vi "main.vi"() -> ()   [LabVIEW 2014]
uses:
  Modules/PmuImpairPlugins/PmuImpairPluginBase_class/TypeDefs/clImpairConfig.ctl
  Framework/FrontPanel/TypeDefs/clEventConfig.ctl
  Framework/FrontPanel/TypeDefs/clFrontPanelControlRefs.ctl
  Framework/FrontPanel/TypeDefs/clFrontPanelButtonRefs.ctl
  Framework/Bus_class/Public/TypeDefs/clBusData.ctl
  Modules/EventPlugins/EventPluginBaseClass/TypeDefs/clEvtReportArray.ctl
  Modules/EventPlugins/EventPluginBaseClass/TypeDefs/clEvtReport.ctl
  Modules/EventPlugins/EventPluginBaseClass/TypeDefs/dblEvtSignalArray.ctl
  Modules/NetworkImpairmentModule/PublicAPI/Arguments/Broadcasts/dblNetworkTime.ctl
  Modules/NetworkImpairmentModule/PublicAPI/Arguments/Broadcasts/dblPktLoss.ctl
  Modules/FlagImpairModule/PublicAPI/Arguments/Broadcasts/ui32FlagImpairmentArray.ctl
  Modules/OutputToFilePlugins/OutputToFileBasePlugin/Typedefs/PmuCfgOpt.ctl
  Framework/Bus_class/Bus.lvclass/Bus.ctl
  Framework/Config_class/Config.lvclass/Config.ctl
  Modules/EventModule/PublicAPI/Arguments/Broadcasts/clDidInit.ctl
  <userlib>/NIST/ModuleAdminLib/ModuleAdmin/ModuleAdmin.lvclass
  Modules/EventModule/PublicAPI/Arguments/Broadcasts/clStatUpdate.ctl
  Modules/EventModule/PublicAPI/Arguments/Broadcasts/clErrorRpt.ctl
  Modules/EventModule/PublicAPI/Arguments/Requests/clStopArgument.ctl
  Modules/PmuImpairModule/PublicAPI/Arguments/Broadcasts/clDidInit.ctl
  Modules/PmuImpairModule/PublicAPI/Arguments/Broadcasts/clStatUpdate.ctl
  Modules/PmuImpairModule/PublicAPI/Arguments/Broadcasts/clErrorRpt.ctl
  Modules/PmuImpairModule/PublicAPI/Arguments/Requests/clStopArgument.ctl
  Modules/NetworkImpairmentModule/PublicAPI/Arguments/Broadcasts/clDidInit.ctl
  Modules/NetworkImpairmentModule/PublicAPI/Arguments/Broadcasts/clStatUpdate.ctl
  Modules/NetworkImpairmentModule/PublicAPI/Arguments/Broadcasts/clErrorRpt.ctl
  Modules/NetworkImpairmentModule/PublicAPI/Arguments/Requests/clStopArgument.ctl
  Modules/FlagImpairModule/PublicAPI/Arguments/Broadcasts/clDidInit.ctl
  Modules/FlagImpairModule/PublicAPI/Arguments/Broadcasts/clStatUpdate.ctl
  Modules/FlagImpairModule/PublicAPI/Arguments/Broadcasts/clErrorRpt.ctl
  Modules/FlagImpairModule/PublicAPI/Arguments/Requests/clStopArgument.ctl
  Modules/AppModule/PublicAPI/Arguments/Broadcasts/clErrorRpt.ctl
  Framework/Bus_class/Accessors/Read AppModuleID.vi
  Framework/Config_class/Accessors/Read PARTF Root Directory.vi
  <vilib>/Utility/error.llb/Error Cluster From Error Code.vi
  <vilib>/ErrorRing/Error Ring.xnode
  Framework/Config_class/Config.lvclass
  Framework/Framework.lvlib
  <userlib>/NIST/NISTErrorLib/NISTErrorLib.lvlib
  Framework/Bus_class/Bus.lvclass
  Modules/EventModule/EventModule.lvlib
  Modules/PmuImpairModule/PmuImpairModule.lvlib
  Modules/NetworkImpairmentModule/NetworkImpairmentModule.lvlib
  Modules/FlagImpairModule/FlagImpairModule.lvlib
  Modules/EventPlugins/EventPluginBaseClass/EventPluginBaseClass.lvclass
  Modules/OutputToFilePlugins/OutputToFileBasePlugin/OutputToFileBasePlugin.lvclass
  Modules/PmuImpairPlugins/PmuImpairPluginBase_class/PmuImpairPluginBase.lvclass
  TestAutomation/Comms/Comms.lvlib
  Modules/AppModule/AppModule.lvlib
  TestAutomation/LV-PY/LV-PY.lvlib
  Framework/BusController/BusController.lvlib
  Modules/OutputToFileModule/OutputToFileModule.lvlib
  <vilib>/Utility/config.llb/NI_LVConfig.lvlib
panel:
  in  "btnScriptPath":bool
  in  "Monte Carlo Script":string="Default.py"
  in  "btnTestPath":bool
  in  "Test File":string="Default.tst"
  in  "ShowPanels?":bool caption="Show Module Panels?"
  in  "chkLeaveCmdOpen":bool caption="Leave Script Window Open for Debugging"
  in  "btnMonteCarlo":bool
  in  "Output File Type":u16(ring) items=["none", "CSV"]
  in  "btnOutToFileConfig":bool
  in  "btnVisualize":bool
  in  "btnOpen":bool
  in  "btnAppConfig":bool
  in  "Application Type":u16(ring) caption="Application" items=["none", "LSE", "Ringdown"]
  in  "Impairments":T1(tab)
  in  "Sensor Impairment Parameters":string[][](table)
  in  "clImpairConfig":T2={"FilterType"="Hamming", "bPosSeq"=TRUE}
  in  "Sensor Impairment Type":u16(ring)=2 items=["C37.118.1 PMU Behaviour", "C37.118.1 PMU DSP Model", "None", "PMU Sine Model", "User Impair Example 1"]
  in  "Network Impairment Type":u16(ring)=1 items=["Network Impairment", "None"]
  in  "Network Impairment Parameters":string[][](table)
  in  "Status Impairment Parameters":string[][](table)
  in  "Status Impairment Type":u16(ring)=2 items=["C37.118.2 PMU Data Transmission", "IEC61850 PMU", "None"]
  in  "Bus Number":u8(ring)
  in  "btnUpdateBus":bool
  in  "btnRemoveBus":bool
  in  "btnAbortMonteCarlo":bool
  in  "btnAddBus":bool
  in  "btnExit":bool
  in  "btnSingleRun":bool
  in  "End Time":dbl=5.0
  in  "Start Time":dbl
  in  "Event Configuration":T3={"UTC Time 0"=timestamp(0 s since 1904-01-01), "Nominal Frequency"=60, "Reporting Rate"=60, "Fsamp"=960, "PosSeq"=TRUE} {"Reporting Rate" items=["10 FPS"=10, "12 FPS"=12, "15 FPS"=15, "20 FPS"=20, "30 FPS"=30, "60 FPS"=60]; "Nominal Frequency" items=["50 Hz"=50, "60 Hz"=60]}
  in  "Event Type":u16(ring) items=["C37.118.1", "Event From CSV", "IEEEBusSystem", "Ringdown", "User1"]
  in  "btnSave":bool
  in  "Event Parameters":string[][](table)=[["70", "70", "70", "20", "20", "20"], ["60", "60", "60", "60", "60", "60"], ["0", "-120", "120", "0", "-120", "120"], ["0", "0", "0", "0", "0", "0"], ["0", "0", "0", "0", "0", "0"], ["0", "0", "0", "0", "0", "0"], ["0", "0", "0", "0", "0", "0"], ["0", "0", "0", "0", "0", "0"], ["0", "0", "0", "0", "0", "0"], ["0", "0", "0", "0", "0", "0"], ["0", "0", "0", "0", "0", "0"], ["0", "0", "0", "0", "0", "0"], ["0", "0", "0", "0", "0", "0"]]
  out "Number of Buses":u8=1 min=1
  in  "btnSettings":bool
  # "The transformer impairment tab will be hidden until\nthe transformer impairment is implemented"
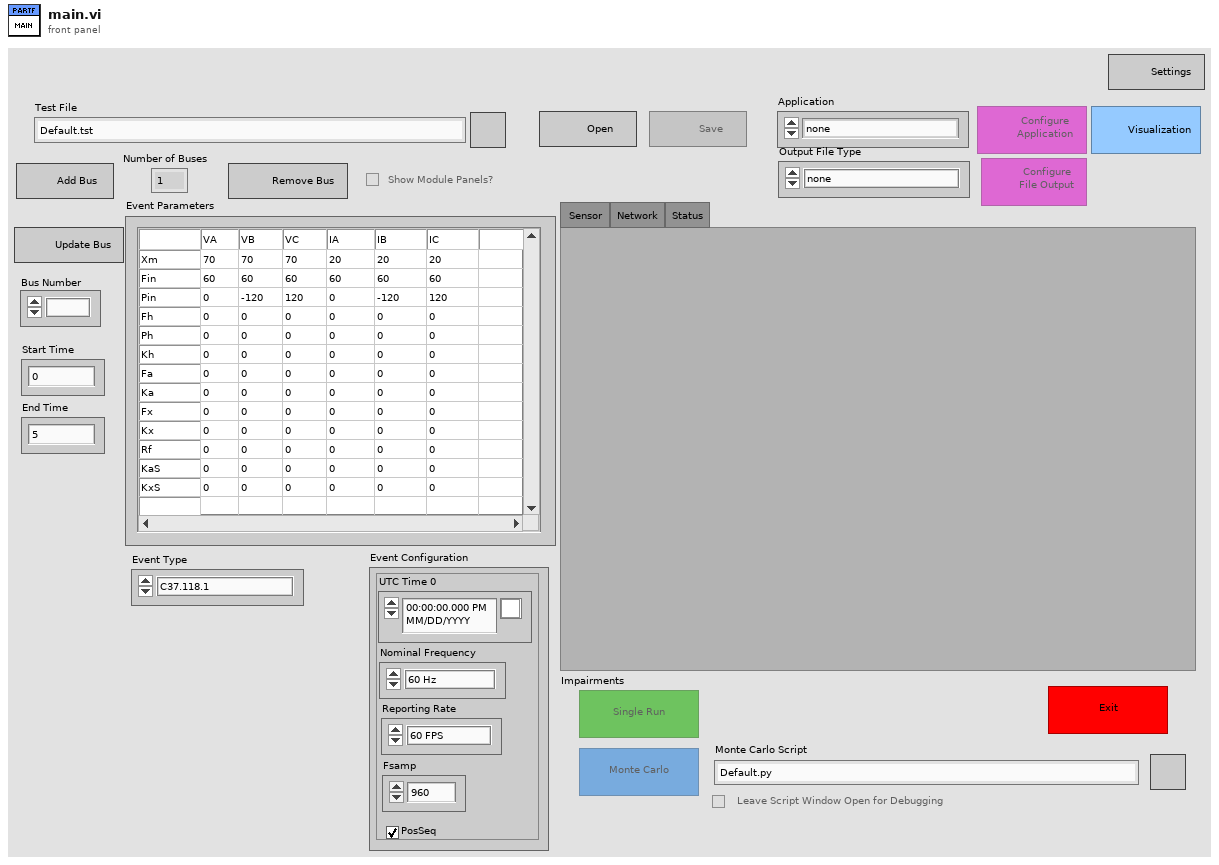
[diagram p1: front panel]
types:
  T1 = enum32{"Transformers", "Sensor ", "Network", "Status"}
  T2 = typedef "PmuImpairPlugins.lvlib/PmuImpairPluginBase.lvclass/clImpairConfig.ctl" = cluster{"FilterType":string, "bPosSeq":bool}
  T3 = typedef "Framework.lvlib/clEventConfig.ctl" = cluster{"UTC Time 0":timestamp, "Nominal Frequency":u16, "Reporting Rate":u16, "Fsamp":u32, "PosSeq":bool}
  T4 = typedef "Framework.lvlib/clFrontPanelButtonRefs.ctl" = cluster{"SaveRef":refnum<vi>, "SingleRunRef":refnum<vi>, "MonteCarloRef":refnum<vi>, "AppConfigRef":refnum<vi>, "chkScriptWindowRef":refnum<vi>, "btnOutToFileConfig":refnum<vi>, "AppTypeRef":refnum<vi>, "chkShowPanel":refnum<vi>}
  T5 = typedef "Framework.lvlib/clFrontPanelControlRefs.ctl" = cluster{"TestFilePathRef":refnum<vi>, "BusNumberRef":refnum<vi>, "NumberOfBusesRef":refnum<vi>, "EvtTypeRef":refnum<vi>, "EvtParamsRef":refnum<vi>, "EvtConfigRef":refnum<vi>, "StartTimeRef":refnum<vi>, "EndTimeRef":refnum<vi>, "PmuImpairTypeRef":refnum<vi>, "PmuImpairParamsRef":refnum<vi>, "NetImpairParamsRef":refnum<vi>, "FlagImpairTypeRef":refnum<vi>, "FlagImpairParamsRef":refnum<vi>, "NetImpairTypeRef":refnum<vi>, "OutputFileType":refnum<vi>, "PmuImpairConfigRef":refnum<vi>, "AppTypeRef":refnum<vi>, "ScriptPathRef":refnum<vi>, "ShowPanels?":refnum<vi>}
  T6 = typedef "EventModule.lvlib/clBroadcastEvents.ctl" = cluster{"DidInit":refnum<user-event>, "StatusUpdate":refnum<user-event>, "ErrorReport":refnum<user-event>, "DidStop":refnum<user-event>, "ReadEvtConfig":refnum<user-event>, "ReadTimeArray":refnum<user-event>, "ReadEvtParams":refnum<user-event>, "GetEvtReportArray":refnum<user-event>, "ReadPathToPlugin":refnum<user-event>, "GetEvtSignal":refnum<user-event>, "ReadBusNumber":refnum<user-event>}
  T7 = typedef "PmuImpairModule.lvlib/clBroadcastEvents.ctl" = cluster{"DidInit":refnum<user-event>, "StatusUpdate":refnum<user-event>, "ErrorReport":refnum<user-event>, "DidStop":refnum<user-event>, "ImpairConfig":refnum<user-event>, "ImpairParams":refnum<user-event>, "ImpairReports":refnum<user-event>, "PathToPlugin":refnum<user-event>, "BusNumber":refnum<user-event>}
  T8 = typedef "NetworkImpairmentModule.lvlib/clBroadcastEvents.ctl" = cluster{"DidInit":refnum<user-event>, "StatusUpdate":refnum<user-event>, "ErrorReport":refnum<user-event>, "DidStop":refnum<user-event>, "ReadNetImpParams":refnum<user-event>, "ReadLossThreshold":refnum<user-event>, "GetNetworkTime":refnum<user-event>, "GetPktLoss":refnum<user-event>, "ReadPathToPlugin":refnum<user-event>}
  T9 = typedef "FlagImpairModule.lvlib/clBroadcastEvents.ctl" = cluster{"DidInit":refnum<user-event>, "StatusUpdate":refnum<user-event>, "ErrorReport":refnum<user-event>, "DidStop":refnum<user-event>, "ReadFlagImpairConfig":refnum<user-event>, "ReadPluginINIFilePath":refnum<user-event>, "ReadFlagImpairParams":refnum<user-event>, "ReadTimeArray":refnum<user-event>, "GetFlagImpairment":refnum<user-event>}
  T10 = typedef "AppModule.lvlib/clBroadcastEvents.ctl" = cluster{"DidInit":refnum<user-event>, "StatusUpdate":refnum<user-event>, "ErrorReport":refnum<user-event>, "DidStop":refnum<user-event>, "PathToINI":refnum<user-event>, "InputData":refnum<user-event>, "OutputData":refnum<user-event>, "BcAppInfo":refnum<user-event>, "ConfigData":refnum<user-event>}
  T11 = typedef "OutputToFileModule.lvlib/clBroadcastEvents.ctl" = cluster{"DidInit":refnum<user-event>, "StatusUpdate":refnum<user-event>, "ErrorReport":refnum<user-event>, "DidStop":refnum<user-event>, "PathToPlugin":refnum<user-event>, "PmuConfig":refnum<user-event>, "OutputPath":refnum<user-event>}
  T12 = typedef "Framework.lvlib/clRequestEvents.ctl" = cluster{"StopRequest":refnum<user-event>}
  T13 = typedef "EventModule.lvlib/clDidInit.ctl" = cluster{"Init?":bool, "ModuleAdmin":refnum<class "ModuleAdmin.lvclass">}
  T14 = typedef "EventModule.lvlib/clStatUpdate.ctl" = cluster{"Status":string}
  T15 = typedef "EventModule.lvlib/clErrorRpt.ctl" = cluster{"error":errorcluster, "AdditionalInfo":string}
  T16 = typedef "EventModule.lvlib/clStopArgument.ctl" = cluster{"Exit via Stop Module Req?":bool, "Wait for Module to stop?":bool, "ModuleAdmin":refnum<class "ModuleAdmin.lvclass">}
  T17 = typedef "PmuImpairModule.lvlib/clDidInit.ctl" = cluster{"Init?":bool, "ModuleAdmin":refnum<class "ModuleAdmin.lvclass">}
  T18 = typedef "PmuImpairModule.lvlib/clStatUpdate.ctl" = cluster{"Status":string}
  T19 = typedef "PmuImpairModule.lvlib/clErrorRpt.ctl" = cluster{"error":errorcluster, "AdditionalInfo":string}
  T20 = typedef "PmuImpairModule.lvlib/clStopArgument.ctl" = cluster{"Exit via Stop Module Req?":bool, "Wait for Module to stop?":bool, "ModuleAdmin":refnum<class "ModuleAdmin.lvclass">}
  T21 = typedef "NetworkImpairmentModule.lvlib/clDidInit.ctl" = cluster{"Init?":bool, "ModuleAdmin":refnum<class "ModuleAdmin.lvclass">}
  T22 = typedef "NetworkImpairmentModule.lvlib/clStatUpdate.ctl" = cluster{"Status":string}
  T23 = typedef "NetworkImpairmentModule.lvlib/clErrorRpt.ctl" = cluster{"error":errorcluster, "AdditionalInfo":string}
  T24 = typedef "NetworkImpairmentModule.lvlib/clStopArgument.ctl" = cluster{"Exit via Stop Module Req?":bool, "Wait for Module to stop?":bool, "ModuleAdmin":refnum<class "ModuleAdmin.lvclass">}
  T25 = typedef "FlagImpairModule.lvlib/clDidInit.ctl" = cluster{"Init?":bool, "ModuleAdmin":refnum<class "ModuleAdmin.lvclass">}
  T26 = typedef "FlagImpairModule.lvlib/clStatUpdate.ctl" = cluster{"Status":string}
  T27 = typedef "FlagImpairModule.lvlib/clErrorRpt.ctl" = cluster{"error":errorcluster, "AdditionalInfo":string}
  T28 = typedef "FlagImpairModule.lvlib/clStopArgument.ctl" = cluster{"Exit via Stop Module Req?":bool, "Wait for Module to stop?":bool, "ModuleAdmin":refnum<class "ModuleAdmin.lvclass">}
  T29 = typedef "AppModule.lvlib/clErrorRpt.ctl" = cluster{"error":errorcluster, "AdditionalInfo":string}
  T30 = typedef "Framework.lvlib/clFrameworkData.ctl" = cluster{"EvtINIFilePaths":path[], "BusClassInstances":refnum<class "Bus.lvclass">[], "PmuImpairINIFilePaths":path[], "FlagImpairINIFilePaths":path[], "NetImpairINIFilePaths":path[], "OutputToFileINIFilePaths":path[], "AppINIFilePaths":path[], "AppModuleID":i32, "OutputToFileID":i32}
  T31 = cluster{"EvtBroadcastEvents":T6, "PmuBroadcastEvents":T7, "NetBroadcastEvents":T8, "FlagImpairBroadcast":T9}
  T32 = typedef "Bus_class.lvlib/Bus.lvclass/clBusData.ctl" = cluster{"BusNumber":u8, "EvtPluginINIFilePath":path, "EvtParams":string[][], "EvtConfig":T3, "Start Time":dbl, "End Time":dbl, "PmuImpairPluginINIFilePath":path, "PmuImpairParams ":string[][], "PmuImpairConfig":T2, "NetImpPluginINIFilePath":path, "NetImpParams":string[][], "FlagImpPluginINIFilePath":path, "FlagImpParams":string[][], "EvtReportArray":T33, "EventSignalArray":T35, "ImpairReportArray":T33, "NetworkTime":T36, "PktLoss":T37, "FlagImpArray":T38, "OutputToFilePluginINIFilePath":path, "Output File Path":path, "clConfigOptions":T39, "AppPluginINIFilePath":path, "AppConfig":variant, "AppOutput":variant}
  T33 = typedef "EventPlugins.lvlib/EventPluginBaseClass.lvclass/clEvtReportArray.ctl" = T34[]
  T34 = typedef "EventPlugins.lvlib/EventPluginBaseClass.lvclass/clEvtReport.ctl" = cluster{"Timestamp":dbl, "Synx":cdb[], "Freq":dbl, "ROCOF":dbl, "ID":i16}
  T35 = typedef "EventPlugins.lvlib/EventPluginBaseClass.lvclass/dblEvtSignalArray.ctl" = dbl[][]
  T36 = typedef "NetworkImpairmentModule.lvlib/dblNetworkTime.ctl" = dbl[]
  T37 = typedef "NetworkImpairmentModule.lvlib/dblPktLoss.ctl" = dbl[]
  T38 = typedef "FlagImpairModule.lvlib/ui32FlagImpairmentArray.ctl" = u32[]
  T39 = typedef "OutputToFilePlugins.lvlib/OutputToFileBasePlugin.lvclass/PmuCfgOpt.ctl" = cluster{"TIME_BASE":u64, "STN":string, "IDCODE":u16, "rdoPolRect":enum32{"Rectangular", "Polar"}, "rdoFloatInt":enum32{"Float", "Integer"}, "PHUNIT":u64, "rdoFreqDfreq":enum32{"Float", "Integer"}, "CHNAM":string[], "chkCfg2Prefix":bool}
  T40 = typedef "NI_LVConfig.lvlib/Config Data RefNum.ctl" = refnum<k1>
  T41 = typedef "AppModule.lvlib/BC_AppInfo.ctl" = cluster{"QueName":string, "BCRegRef":refnum<data-value>}
  T42 = typedef "Framework.lvlib/Config.lvclass/RootDir.ctl" = cluster{"pathRootDir":path, "btnOutPath":bool, "OutDir":string, "btnOpenOutputDir":bool, "ScriptDir":string, "btnOpenScriptDir":bool, "TestDir":string, "btnOpenTestDir":bool}
  T43 = enum8{"Enabled", "Disabled", "Disabled and Grayed Out"}
  T44 = typedef "Framework.lvlib/QueRef.ctl" = refnum<queue>
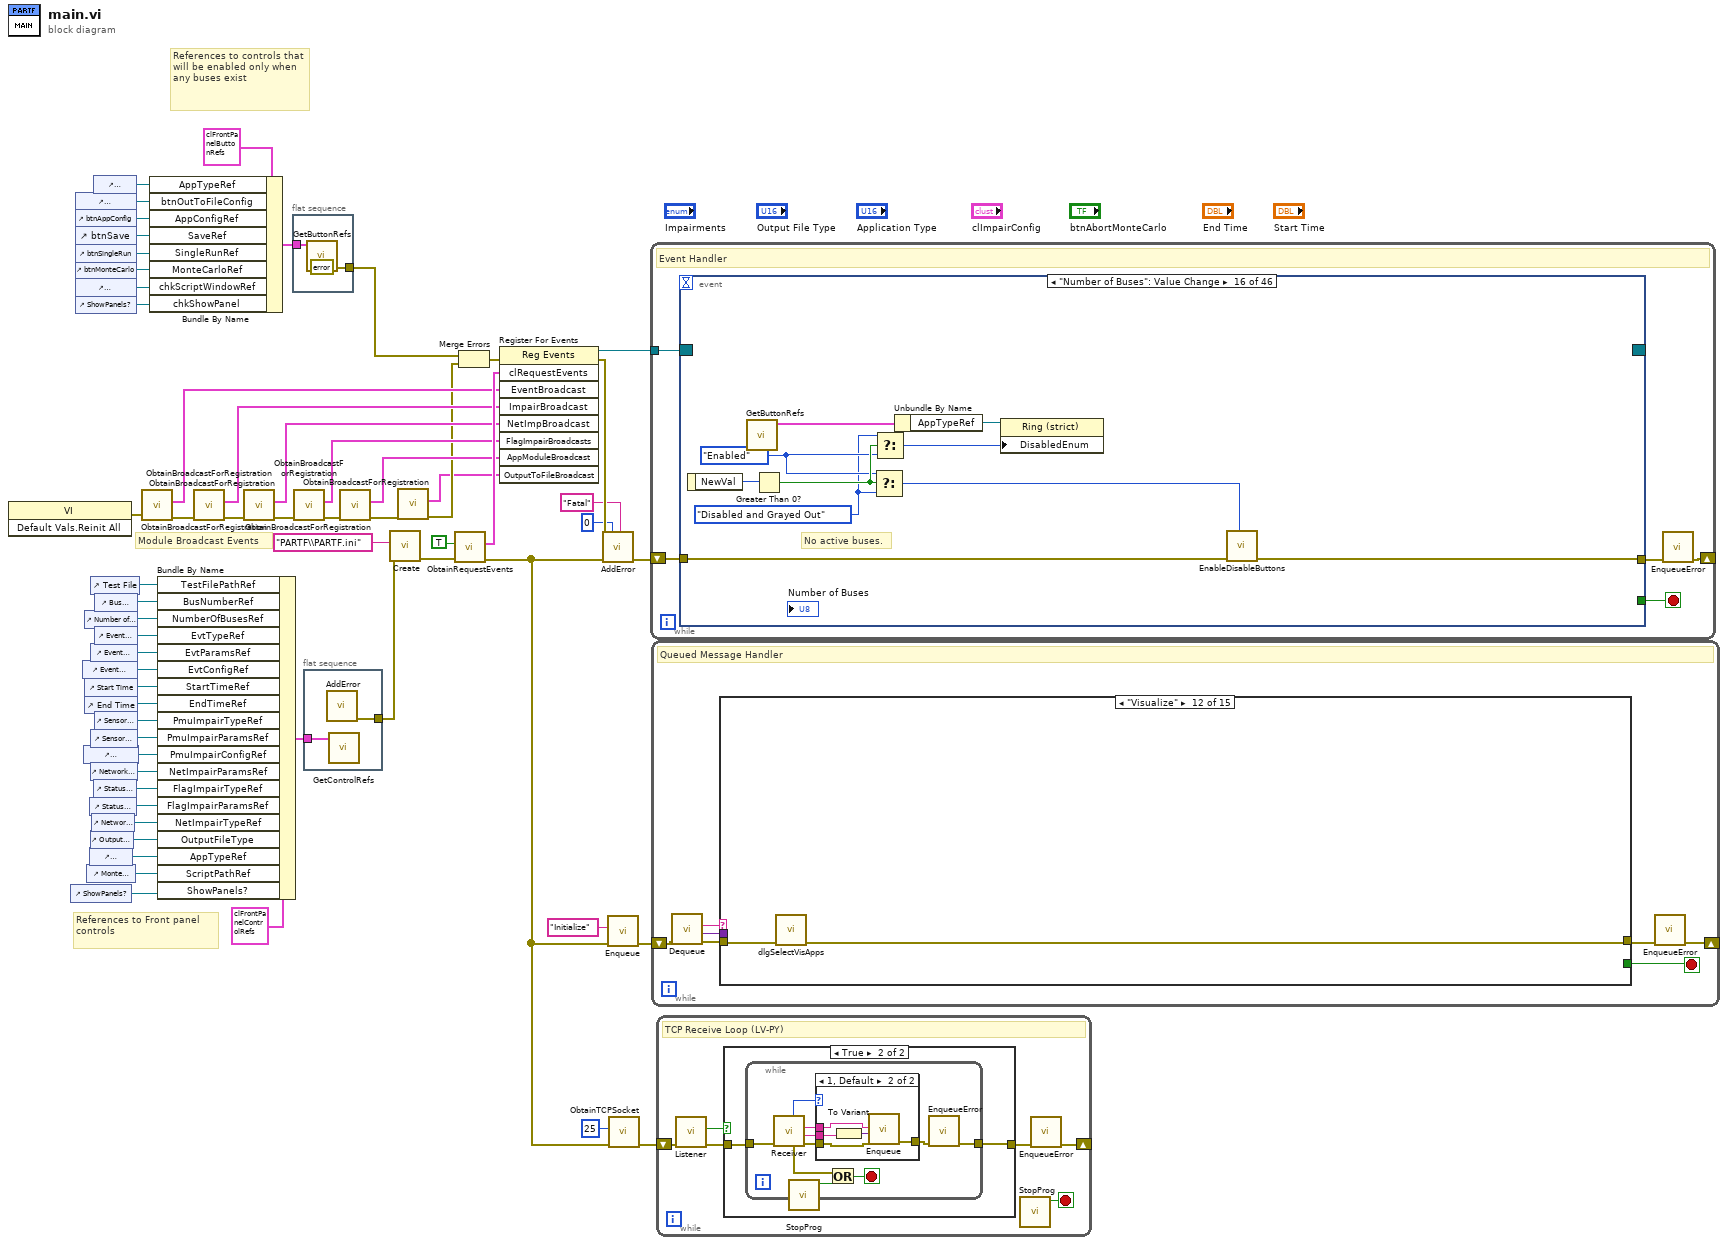
[diagram p0: block diagram]
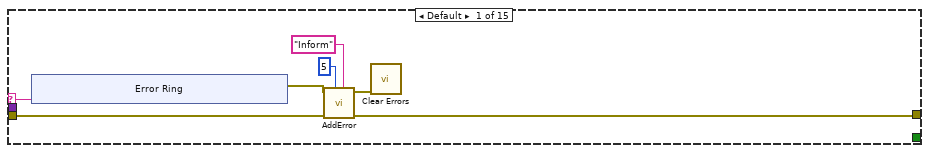
[diagram p4: hidden frame]
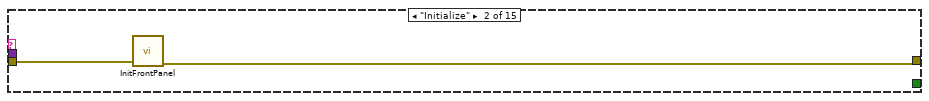
[diagram p5: hidden frame]
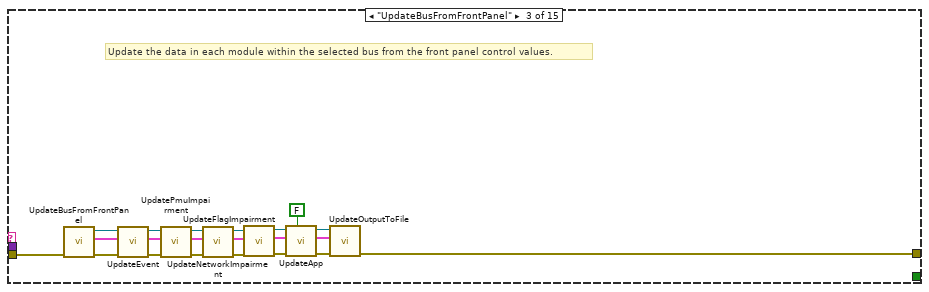
[diagram p6: hidden frame]
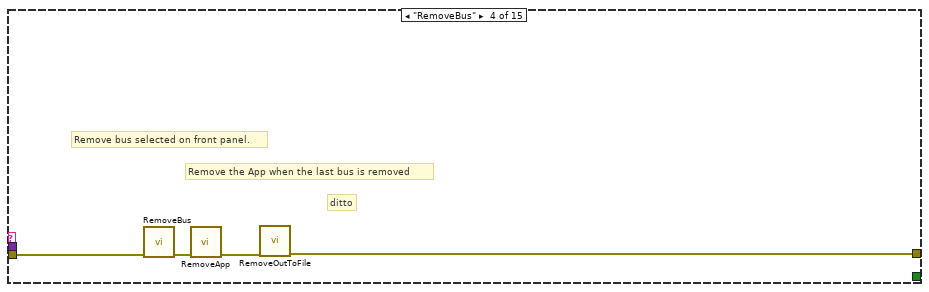
[diagram p7: hidden frame]
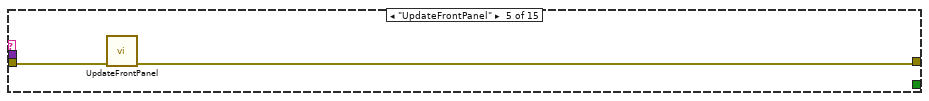
[diagram p8: hidden frame]
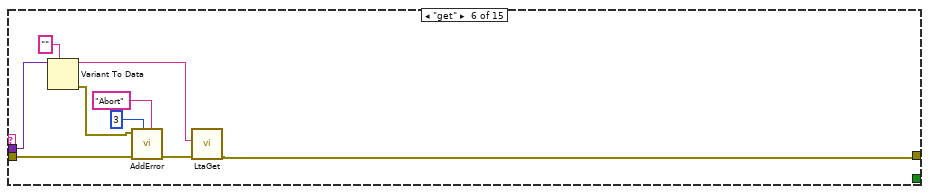
[diagram p9: hidden frame]
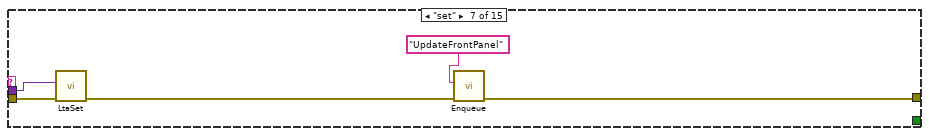
[diagram p10: hidden frame]
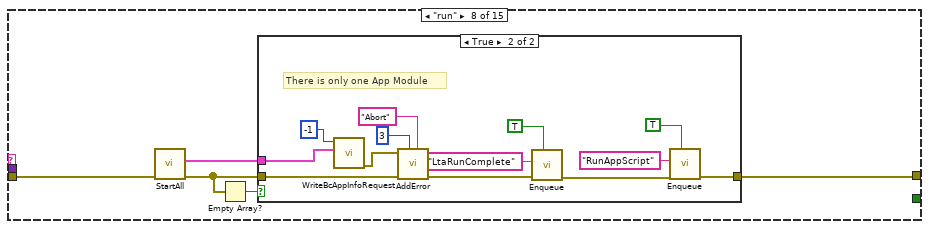
[diagram p11: hidden frame]
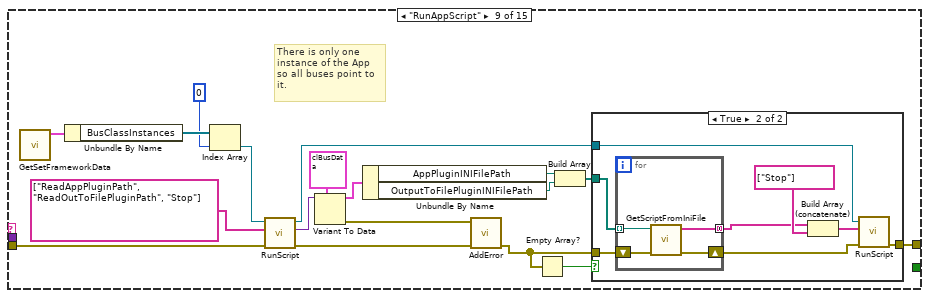
[diagram p13: hidden frame]
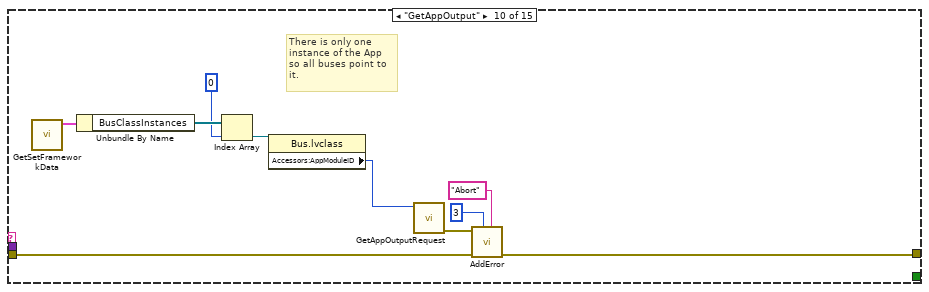
[diagram p15: hidden frame]
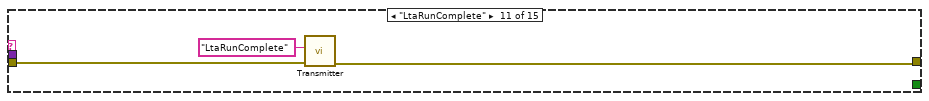
[diagram p16: hidden frame]
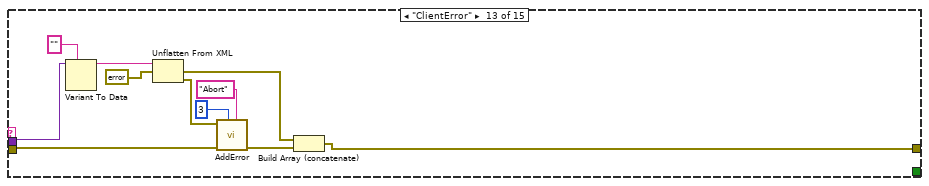
[diagram p17: hidden frame]
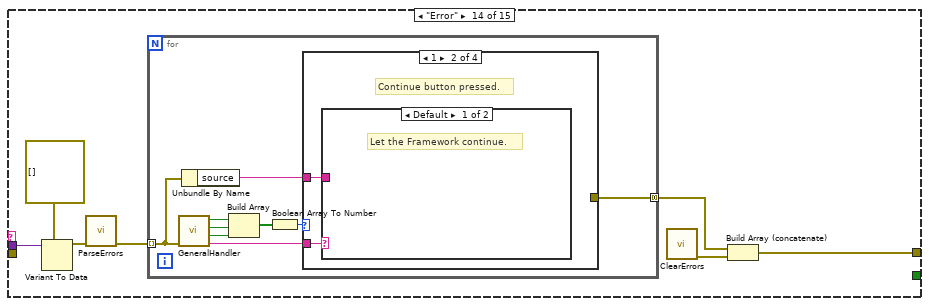
[diagram p18: hidden frame]
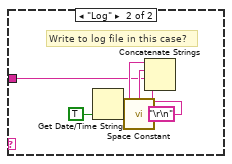
[diagram p20: hidden frame]
diagram:
  # "References to Front panel controls"
  # "Module Broadcast Events"
  # "References to controls that will be enabled only when any buses exist"
  n1 = invoke class="VI" method="Default Vals.Reinit All"() -> (error out=w4:errorcluster)  [unwired: 3 in, 2 out]
  n2 = control-ref of="ShowPanels?"() -> (w10:refnum<vi>)
  n3 = control-ref of="btnOutToFileConfig"() -> (w17:refnum<vi>)
  n4 = control-ref of="btnAppConfig"() -> (w21:refnum<vi>)
  n5 = control-ref of="btnSave"() -> (w46:refnum<vi>)
  n6 = control-ref of="btnSingleRun"() -> (w45:refnum<vi>)
  n7 = control-ref of="btnMonteCarlo"() -> (w44:refnum<vi>)
  n8 = control-ref of="chkLeaveCmdOpen"() -> (w20:refnum<vi>)
  n9 = control-ref of="ShowPanels?"() -> (w9:refnum<vi>)
  n10 = control-ref of="Event Configuration"() -> (w37:refnum<vi>)
  n11 = control-ref of="clImpairConfig"() -> (w24:refnum<vi>)
  n12 = control-ref of="Number of Buses"() -> (w34:refnum<vi>)
  n13 = control-ref of="Start Time"() -> (w33:refnum<vi>)
  n14 = control-ref of="End Time"() -> (w32:refnum<vi>)
  n15 = control-ref of="Monte Carlo Script"() -> (w12:refnum<vi>)
  n16 = control-ref of="Status Impairment Parameters"() -> (w40:refnum<vi>)
  n17 = control-ref of="Application Type"() -> (w13:refnum<vi>)
  n18 = control-ref of="Test File"() -> (w39:refnum<vi>)
  n19 = control-ref of="Event Parameters"() -> (w36:refnum<vi>)
  n20 = control-ref of="Sensor Impairment Parameters"() -> (w54:refnum<vi>)
  n21 = control-ref of="Network Impairment Parameters"() -> (w48:refnum<vi>)
  n22 = control-ref of="Output File Type"() -> (w25:refnum<vi>)
  n23 = control-ref of="Network Impairment Type"() -> (w26:refnum<vi>)
  n24 = control-ref of="Application Type"() -> (w11:refnum<vi>)
  n25 = control-ref of="Status Impairment Type"() -> (w41:refnum<vi>)
  n26 = control-ref of="Bus Number"() -> (w38:refnum<vi>)
  n27 = control-ref of="Event Type"() -> (w35:refnum<vi>)
  n28 = control-ref of="Sensor Impairment Type"() -> (w31:refnum<vi>)
  n29 = call "ObtainBroadcastForRegistration.vi"("error in (no error)"=w4) -> ("error out"=w52:errorcluster, "EventBroadcast"=w53:T6)  [unwired: 9 in]
  n30 = Bundle By Name(cluster=T4 {"SaveRef"=refnum, "SingleRunRef"=refnum, "MonteCarloRef"=refnum, "AppConfigRef"=refnum, "chkScriptWindowRef"=refnum, "btnOutToFileConfig"=refnum, "AppTypeRef"=refnum, "chkShowPanel"=refnum} ("clFrontPanelButtonRefs"), "AppTypeRef"=w11, "btnOutToFileConfig"=w17, "AppConfigRef"=w21, "SaveRef"=w46, "SingleRunRef"=w45, "MonteCarloRef"=w44, "chkScriptWindowRef"=w20, "chkShowPanel"=w9) -> (w3:T4)
  n31 = Bundle By Name(cluster=T5 {"TestFilePathRef"=refnum, "BusNumberRef"=refnum, "NumberOfBusesRef"=refnum, "EvtTypeRef"=refnum, "EvtParamsRef"=refnum, "EvtConfigRef"=refnum, "StartTimeRef"=refnum, "EndTimeRef"=refnum, "PmuImpairTypeRef"=refnum, "PmuImpairParamsRef"=refnum, "NetImpairParamsRef"=refnum, "FlagImpairTypeRef"=refnum, "FlagImpairParamsRef"=refnum, "NetImpairTypeRef"=refnum, "OutputFileType"=refnum, "PmuImpairConfigRef"=refnum, "AppTypeRef"=refnum, "ScriptPathRef"=refnum, "ShowPanels?"=refnum} ("clFrontPanelControlRefs"), "TestFilePathRef"=w39, "BusNumberRef"=w38, "NumberOfBusesRef"=w34, "EvtTypeRef"=w35, "EvtParamsRef"=w36, "EvtConfigRef"=w37, "StartTimeRef"=w33, "EndTimeRef"=w32, "PmuImpairTypeRef"=w31, "PmuImpairParamsRef"=w54, "PmuImpairConfigRef"=w24, "NetImpairParamsRef"=w48, "FlagImpairTypeRef"=w41, "FlagImpairParamsRef"=w40, "NetImpairTypeRef"=w26, "OutputFileType"=w25, "AppTypeRef"=w13, "ScriptPathRef"=w12, "ShowPanels?"=w10) -> (w8:T5)
  n32 = call "ObtainBroadcastForRegistration.vi"("error in (no error)"=w52) -> ("error out"=w50:errorcluster, "ImpairBroadcast"=w51:T7)  [unwired: 9 in]
  n33 = call "ObtainBroadcastForRegistration.vi"("error in (no error)"=w50) -> ("error out"=w43:errorcluster, "NetImpBroadcast"=w49:T8)  [unwired: 9 in]
  n34 = flat-sequence {
    tunnel: w3 -> [w63]
    tunnel: [errorcluster {"status"=FALSE, "code"=0, "source"=""} ("error constant")] -> w1
    frame #0 {
      n35 = call "GetButtonRefs.vi"("BtnRefs"=w63) -> ()  [unwired: 10 in, 1 out]
    }
  }
  n36 = call "ObtainBroadcastForRegistration.vi"("error in (no error)"=w43) -> ("error out"=w19:errorcluster, "FlagImpairBroadcasts"=w42:T9)  [unwired: 9 in]
  n37 = flat-sequence {
    tunnel: w8 -> [w64]
    tunnel: [w65] -> w6
    frame #0 {
      n38 = call <userlib>:"AddError.vi"() -> ("ErrorArray"=w65:errorcluster[])  [unwired: 10 in, 1 out]
      n39 = call "GetControlRefs.vi"("clControlRefs In"=w64) -> ()  [unwired: 10 in, 1 out]
    }
  }
  n40 = call "ObtainBroadcastForRegistration.vi"("error in (no error)"=w19) -> ("error out"=w16:errorcluster, "AppModuleBroadcast"=w18:T10)  [unwired: 9 in]
  n41 = call "Create.vi"("ErrorArray"=w6, "name or relative path"="PARTF\\PARTF.ini") -> ("ErrorArray"=w5:errorcluster[])  [unwired: 8 in, 1 out]
  n42 = call "ObtainBroadcastForRegistration.vi"("error in (no error)"=w16) -> ("error out"=w15:errorcluster, "OutputToFileBroadcast"=w14:T11)  [unwired: 9 in]
  n43 = call "ObtainRequestEvents.vi"("ErrorArray In"=w5, "CreateNew (F)"=TRUE) -> ("ErrorArray Out"=w55:errorcluster[], "clRequestEvents"=w59:T12)  [unwired: 8 in]
  n44 = Merge Errors(w1, w15) -> (w2:errorcluster)
  n45 = register-events(error in=w2, w59, w53, w51, w49, w42, w18, w14) -> (reference out=w58:refnum<event-registration>, error out=w29:errorcluster)  [unwired: 1 in]
  n46 = call <userlib>:"AddError.vi"("Severity"="Fatal" ("String"), "Priority"=u8 0, "ErrorArray"=w55, "error in (no error)"=w29) -> ("ErrorArray"=w30:errorcluster[])  [unwired: 6 in, 1 out]
  n47 = call "Enqueue.vi"("ErrorArray"=w5, "Msg"="Initialize") -> ("ErrorArray"=w61:errorcluster[])  [unwired: 9 in]
  n48 = call "ObtainTCPSocket.vi"("ErrorArray"=w5, "timeout"=25) -> ("ErrorArray"=w23:errorcluster[])  [unwired: 8 in, 1 out]
  n49 = while {
    shift-right: [w67] -> _
    shift-left: w30 -> [w69]
    tunnel: w58 -> [w66]
    stop <- w70 stop-if-true
    # "Event Handler"
    n50 = event shown="[15] \"Number of Buses\": Value Change" {
      selector: w66 -> [_ _ _ w125 _ _ _ w164 _ _ _ _ _ _ _ _ _ _ _ _ _ _ _ _ _ _ _ _ _ _ _ _ _ _ _ _ _ _ _ _ _ _ _ _ _ _]
      dyn-events: [_ _ _ w124 _ _ _ w163 _ _ _ _ _ _ _ _ _ _ _ _ _ _ _ _ _ _ _ _ _ _ _ _ _ _ _ _ _ _ _ _ _ _ _ _ _ _] -> _
      timeout: _ -> [_ _ _ _ _ _ _ _ _ _ _ _ _ _ _ _ _ _ _ _ _ _ _ _ _ _ _ _ _ _ _ _ _ _ _ _ _ _ _ _ _ _ _ _ _ _]
      tunnel: [TRUE _ _ _ _ _ _ _ _ _ _ _ _ _ _ _ _ _ _ _ _ _ _ _ _ _ _ _ TRUE _ _ _ _ _ _ _ _ _ _ _ _ _ _ _ _ _] -> w70
      tunnel: w69 -> [w78 w81 w86 w115 w138 w148 w153 w165 w221 w225 _ w252 w276 _ w305 w315 w318 w322 w324 w326 w328 w331 _ _ w350 w355 w360 w363 w366 w374 w395 w409 w420 w443 w462 w478 w489 w509 w530 w548 w556 w577 w597 w615 w625 w646]
      tunnel: [w77 w80 w85 w96 w139 w151 w152 w162 w220 w226 _ w255 w279 w301 w304 w314 w317 w321 w323 w325 w327 w330 _ _ w349 w351 w356 w362 w365 w373 w393 w410 w422 w442 w464 w479 w491 w507 w529 w546 w557 w576 w599 w617 w626 w648] -> w68
      event "btnExit": Value Change {
        n51 = event-data() -> ()  [unwired: 1 in, 1 out]
        n52 = call "RemoveBus.vi"("Remove All? (F)"=TRUE, "ErrorArray In"=w78) -> ("ErrorArray Out"=w73:errorcluster[])  [unwired: 9 in]
        n53 = call "RemoveApp.vi"("ErrorArray In"=w73) -> ("ErrorArray Out"=w71:errorcluster[])  [unwired: 10 in]
        n54 = call "RemoveOutToFile.vi"("ErrorArray In"=w71) -> ("ErrorArray Out"=w72:errorcluster[])  [unwired: 10 in]
        n55 = call "Enqueue.vi"("Priority (f)"=TRUE, "ErrorArray"=w72, "Msg"="Stop") -> ("ErrorArray"=w77:errorcluster[])  [unwired: 8 in]
      }
      event "btnSettings": Value Change {
        n56 = event-data() -> ()  [unwired: 1 in, 1 out]
        n57 = call "Settings.vi"("ErrorArray"=w81) -> ("ErrorArray"=w80:errorcluster[])  [unwired: 10 in]
      }
      event "btnOutToFileConfig": Value Change {
        n58 = event-data() -> ()  [unwired: 1 in, 1 out]
        n59 = call "GetSetFrameworkData.vi"() -> ("clFrameworkData Out"=w88:T30)  [unwired: 11 in]
        n60 = Unbundle By Name(w88) -> ("OutputToFileID"=w87:i32)
        n61 = call "OpenConfigRequest.vi"("ModuleID"=w87) -> ("error out"=w84:errorcluster)  [unwired: 10 in]
        n62 = call <userlib>:"AddError.vi"("Severity"="Inform", "Priority"=u8 4, "ErrorArray"=w86, "error in (no error)"=w84) -> ("ErrorArray"=w85:errorcluster[])  [unwired: 6 in, 1 out]
      }
      event "btnAddBus": Value Change {
        n63 = event-data() -> ()  [unwired: 1 in, 1 out]
        n64 = property on="ShowPanels?" class="Bool (strict)"() -> ("Value"=w89:bool)  [unwired: 2 in, 2 out]
        n65 = call "Create.vi"("Error In"=w115) -> ("Error Out"=w120:errorcluster[], "Bus out"=w119:refnum<class "Bus.lvclass">)  [unwired: 9 in]
        n66 = call "AddBus.vi"("ShowPanels?"=w89, "ErrorArray In"=w120, "BusClass In"=w119) -> ("ErrorArray Out"=w123:errorcluster[], "UserEvents"=w117:T31, "BusClass Out"=w122:refnum<class "Bus.lvclass">)  [unwired: 6 in]
        n67 = call "AddApp.vi"("ErrorArray In"=w123, "BusClass In"=w122) -> ("ErrorArray Out"=w95:errorcluster[], "clBroadcastEvents"=w121:T10, "BusClass Out"=w93:refnum<class "Bus.lvclass">)  [unwired: 7 in]
        n68 = call "AddOutToFile.vi"("ErrorArray In"=w95, "BusClass In"=w93) -> ("ErrorArray Out"=w94:errorcluster[], "clBroadcastEvents"=w91:T11, "BusClass Out"=w92:refnum<class "Bus.lvclass">)  [unwired: 7 in]
        n69 = Empty Array?(array=w94) -> (empty?=w116:bool)
        n70 = call "InsertBus.vi"("ErrorArray In"=w94, "BusClass In"=w92) -> ("ErrorArray Out"=w118:errorcluster[])  [unwired: 8 in, 1 out]
        n71 = case shown="True" w116 {
          tunnel: w121 -> [_ w128]
          tunnel: [w126 w135] -> w124
          tunnel: w117 -> [_ w134]
          tunnel: w125 -> [w126 w129]
          tunnel: w91 -> [_ w127]
          frame False {
          }
          frame True {
            n72 = Unbundle(w134) -> ("EvtBroadcastEvents"=w133:T6, "PmuBroadcastEvents"=w132:T7, "NetBroadcastEvents"=w131:T8, "FlagImpairBroadcast"=w130:T9)
            n73 = register-events(reference=w129, w133, w132, w131, w130, w128, w127) -> (reference out=w135:refnum<event-registration>)  [unwired: 2 in, 1 out]
          }
        }
        n74 = call "UpdateBusFromFrontPanel.vi"("ErrorArray In"=w118) -> ("ErrorArray Out"=w114:errorcluster[], "output cluster"=w113:T32, "Framework.lvlib:Bus.lvclass"=w112:refnum<class "Bus.lvclass">)  [unwired: 8 in]
        n75 = call "UpdateEvent.vi"("ErrorArray In"=w114, "clBusData In"=w113, "Bus.lvclass In"=w112) -> ("ErrorArray Out"=w111:errorcluster[], "clBusData Out"=w110:T32, "Bus.lvclass Out"=w109:refnum<class "Bus.lvclass">)  [unwired: 6 in]
        n76 = call "UpdatePmuImpairment.vi"("ErrorArray In"=w111, "clBusData In"=w110, "Bus.lvclass In"=w109) -> ("ErrorArray Out"=w108:errorcluster[], "clBusData Out"=w107:T32, "Bus.lvclass Out"=w106:refnum<class "Bus.lvclass">)  [unwired: 6 in]
        n77 = call "UpdateNetworkImpairment.vi"("ErrorArray In"=w108, "clBusData In"=w107, "Bus.lvclass In"=w106) -> ("ErrorArray Out"=w105:errorcluster[], "clBusData Out"=w104:T32, "Bus.lvclass Out"=w103:refnum<class "Bus.lvclass">)  [unwired: 6 in]
        n78 = call "UpdateFlagImpairment.vi"("ErrorArray In"=w105, "clBusData In"=w104, "Bus.lvclass In"=w103) -> ("ErrorArray Out"=w101:errorcluster[], "clBusData Out"=w100:T32, "Bus.lvclass Out"=w102:refnum<class "Bus.lvclass">)  [unwired: 6 in]
        n79 = call "UpdateOutputToFile.vi"("ErrorArray In"=w101, "clBusData In"=w100, "Bus.lvclass In"=w102) -> ("ErrorArray Out"=w99:errorcluster[], "clBusData Out"=w98:T32, "Bus.lvclass Out"=w97:refnum<class "Bus.lvclass">)  [unwired: 6 in]
        n80 = call "UpdateApp.vi"("DefaultAppConfig? (f)"=TRUE, "ErrorArray In"=w99, "clBusData in"=w98, "Bus.lvclass"=w97) -> ("ErrorArray Out"=w96:errorcluster[])  [unwired: 5 in, 2 out]
      }
      event "btnRemoveBus": Value Change {
        n81 = event-data() -> ()  [unwired: 1 in, 1 out]
        n82 = call "Enqueue.vi"("Priority (f)"=TRUE, "ErrorArray"=w138, "Msg"="RemoveBus") -> ("ErrorArray"=w139:errorcluster[])  [unwired: 8 in]
      }
      event "ShowPanels?": Value Change {
        w141 = -1 ("ModuleID")
        n83 = event-data() -> ("NewVal"=w140:bool)  [unwired: 1 in]
        n84 = call "ShowPanelRequest.vi"("ShowPanel?"=w140, "ModuleID"=w141) -> ("error out"=w147:errorcluster)  [unwired: 9 in]
        n85 = call "ShowPanelRequest.vi"("error in (no error)"=w147, "ShowPanel?"=w140, "ModuleID"=w141) -> ("error out"=w146:errorcluster)  [unwired: 8 in]
        n86 = call "ShowPanelRequest.vi"("error in (no error)"=w146, "ShowPanel?"=w140, "ModuleID"=w141) -> ("error out"=w145:errorcluster)  [unwired: 8 in]
        n87 = call "ShowPanelRequest.vi"("error in (no error)"=w145, "ShowPanel?"=w140, "ModuleID"=w141) -> ("error out"=w144:errorcluster)  [unwired: 8 in]
        n88 = call "ShowPanelRequest.vi"("error in (no error)"=w144, "ShowPanel"=w140, "ModuleID"=w141) -> ("error out"=w143:errorcluster)  [unwired: 8 in]
        n89 = call "ShowPanelRequest.vi"("error in (no error)"=w143, "ShowPanel"=w140, "Numeric"=w141) -> ("error out"=w142:errorcluster)  [unwired: 8 in]
        n90 = call <userlib>:"AddError.vi"("Severity"="Inform", "Priority"=u8 4, "ErrorArray"=w148, "error in (no error)"=w142) -> ("ErrorArray"=w151:errorcluster[])  [unwired: 6 in, 1 out]
      }
      event "btnUpdateBus": Value Change {
        n91 = event-data() -> ()  [unwired: 1 in, 1 out]
        n92 = call "Enqueue.vi"("Priority (f)"=TRUE, "ErrorArray"=w153, "Msg"="UpdateBusFromFrontPanel") -> ("ErrorArray"=w152:errorcluster[])  [unwired: 8 in]
      }
      event "btnOpen": Value Change {
        # "Remove all open\nbuses. Create array\nof BusClassInstances\n(with set BusNumbers)\nand BusData from \ntest file."
        n93 = event-data() -> ()  [unwired: 1 in, 1 out]
        n94 = call "OpenTestFile.vi"("ErrorArray In"=w165) -> ("ErrorArray Out"=w159:errorcluster[], "BusData"=w161:T32[], "TestFileRef out"=w160:T40)  [unwired: 8 in]
        n95 = Empty Array?(array=w159) -> (empty?=w157:bool)
        n96 = Empty Array?(array=w161) -> (empty?=w158:bool)
        n97 = Compound Arithmetic op=OR(w158, invert w157) -> (w156:bool)
        n98 = case shown="False" w156 {
          tunnel: w161 -> [w173 _]
          tunnel: w159 -> [w184 w218]
          tunnel: w164 -> [w185 w219]
          tunnel: [w183 w219] -> w163
          tunnel: [w179 w218] -> w162
          tunnel: w160 -> [w170 _]
          frame False {
            n99 = for {
              shift-right: [w204] -> w183
              shift-left: w185 -> [w206]
              tunnel: w173 -> [w195] mode=indexing
              shift-right: [w194] -> w172
              shift-left: w184 -> [w199]
              tunnel: [w193] -> w177
              tunnel: [w187] -> w171
              n100 = property on="ShowPanels?" class="Bool (strict)"() -> ("Value"=w186:bool)  [unwired: 2 in, 2 out]
              n101 = call "Create.vi"("Error In"=w199) -> ("Error Out"=w198:errorcluster[], "Bus out"=w197:refnum<class "Bus.lvclass">)  [unwired: 9 in]
              n102 = call "AddBus.vi"("ShowPanels?"=w186, "ErrorArray In"=w198, "BusClass In"=w197) -> ("ErrorArray Out"=w202:errorcluster[], "UserEvents"=w205:T31, "BusClass Out"=w201:refnum<class "Bus.lvclass">)  [unwired: 6 in]
              n103 = call "AddApp.vi"("ErrorArray In"=w202, "BusClass In"=w201) -> ("ErrorArray Out"=w192:errorcluster[], "clBroadcastEvents"=w200:T10, "BusClass Out"=w191:refnum<class "Bus.lvclass">)  [unwired: 7 in]
              n104 = call "AddOutToFile.vi"("ErrorArray In"=w192, "BusClass In"=w191) -> ("ErrorArray Out"=w190:errorcluster[], "clBroadcastEvents"=w188:T11, "BusClass Out"=w189:refnum<class "Bus.lvclass">)  [unwired: 7 in]
              n105 = Empty Array?(array=w190) -> (empty?=w203:bool)
              n106 = call "InsertBus.vi"("ErrorArray In"=w190, "BusClass In"=w189) -> ("ErrorArray Out"=w196:errorcluster[], "BusClass Out"=w187:refnum<class "Bus.lvclass">)  [unwired: 8 in]
              n107 = case shown="True" w203 {
                tunnel: w206 -> [w207 w217]
                tunnel: w205 -> [_ w216]
                tunnel: [w207 w211] -> w204
                tunnel: w200 -> [_ w210]
                tunnel: [_ w209] -> w193
                tunnel: w188 -> [_ w208]
                frame False {
                }
                frame True {
                  n108 = Unbundle(w216) -> ("EvtBroadcastEvents"=w215:T6, "PmuBroadcastEvents"=w214:T7, "NetBroadcastEvents"=w213:T8, "FlagImpairBroadcast"=w212:T9)
                  n109 = register-events(reference=w217, w215, w214, w213, w212, w210, w208) -> (reference out=w211:refnum<event-registration>, error out=w209:errorcluster)  [unwired: 2 in]
                }
              }
              n110 = call "UpdateBusFromFile.vi"("ErrorArray In"=w196, "clBusData"=w195) -> ("ErrorArray Out"=w194:errorcluster[])  [unwired: 8 in, 1 out]
            }
            n111 = call "UpdateAppFromFile.vi"("ErrorArray In"=w172, "TestFileRef In"=w170, "Bus In"=w171) -> ("ErrorArray Out"=w169:errorcluster[], "TestFileRef out"=w168:T40, "Bus Out"=w167:refnum<class "Bus.lvclass">)  [unwired: 6 in]
            n112 = call "UpdateOutToFileFromFile.vi"("ErrorArray In"=w169, "TestFileRef In"=w168, "Bus In"=w167) -> ("ErrorArray Out"=w176:errorcluster[], "refnum out"=w166:T40)  [unwired: 6 in, 1 out]
            n113 = call <vilib>:"Close Config Data.vi"("refnum"=w166) -> ("error out"=w178:errorcluster)  [unwired: 9 in, 1 out]
            n114 = Merge Errors(w177, w178) -> (w174:errorcluster)
            n115 = call <userlib>:"AddError.vi"("Severity"="Inform", "Priority"=u8 4, "ErrorArray"=w176, "error in (no error)"=w174) -> ("ErrorArray"=w175:errorcluster[])  [unwired: 6 in, 1 out]
            n116 = call "Enqueue.vi"("ErrorArray"=w175, "Msg"="UpdateFrontPanel") -> ("ErrorArray"=w179:errorcluster[])  [unwired: 9 in]
          }
          frame True {
          }
        }
      }
      event "btnSave": Value Change {
        # "Save the BusData from all of the open buses in the\nuser-specified test file location.  This overwrites\nexisting files without asking the user if it should.\nIt would be nice to add a dialogue that allows the\nuser to abort the save process if the file already exists\nand they do not want to overwrite."
        n117 = event-data() -> ()  [unwired: 1 in, 1 out]
        n118 = call "SaveTestFile.vi"("ErrorArray In"=w221) -> ("ErrorArray Out"=w220:errorcluster[])  [unwired: 10 in]
      }
      event "btnSingleRun": Value Change {
        n119 = event-data() -> ()  [unwired: 1 in, 1 out]
        n120 = call "StartAll.vi"("Error In"=w225) -> ("Error Out"=w223:errorcluster[], "BC_AppInfo"=w224:T41)  [unwired: 9 in]
        n121 = Empty Array?(array=w223) -> (empty?=w222:bool)
        n122 = case shown="True" w222 {
          tunnel: [w227 w238] -> w226
          tunnel: w223 -> [w227 w234]
          tunnel: w224 -> [_ w232]
          frame False {
          }
          frame True {
            # "There is only one App Module"
            n123 = call "WriteBcAppInfoRequest.vi"("InputData"=w232, "ModuleID"=-1) -> ("error out"=w235:errorcluster)  [unwired: 9 in]
            n124 = call <userlib>:"AddError.vi"("Severity"="Abort", "Priority"=u8 3, "ErrorArray"=w234, "error in (no error)"=w235) -> ("ErrorArray"=w231:errorcluster[])  [unwired: 6 in, 1 out]
            n125 = call "Enqueue.vi"("Priority (f)"=TRUE, "ErrorArray"=w231, "Msg"="RunAppScript") -> ("ErrorArray"=w230:errorcluster[])  [unwired: 8 in]
            n126 = call "Enqueue.vi"("ErrorArray"=w230, "Msg"="GetAppOutput") -> ("ErrorArray"=w238:errorcluster[])  [unwired: 9 in]
          }
        }
      }
      event "btnMonteCarlo": Value Change {
        n127 = event-data() -> ()  [unwired: 1 in, 1 out]
        n128 = call "GetControlRefs.vi"() -> ("clControlRefs Out"=w248:T5)  [unwired: 11 in]
        n129 = call "GetSetConfigClass.vi"() -> ("Ref out"=w247:refnum<class "Config.lvclass">)  [unwired: 11 in]
        n130 = Unbundle By Name(w248) -> ("ScriptPathRef"=w245:refnum<vi>)
        n131 = property class="Config.lvclass"(reference=w247) -> ("Accessors:PARTF Root Directory"=w246:T42)  [unwired: 1 in, 2 out]
        n132 = property class="Str"(reference=w245) -> ("Value"=w241:string)  [unwired: 1 in, 2 out]
        n133 = Unbundle By Name(w246) -> ("pathRootDir"=w243:path, "ScriptDir"=w244:string)
        n134 = Build Path(base path=w243, name or relative path=w244) -> (appended path=w242:path)
        n135 = Build Path(base path=w242, name or relative path=w241) -> (appended path=w240:path)
        n136 = call "RunPython.vi"("keep cmd window open (f)"="chkLeaveCmdOpen", "PathToScript"=w240) -> ()  [unwired: 8 in, 2 out]
      }
      event "btnScriptPath": Value Change {
        w259 = "*.py" ("pattern (all files)")
        n137 = event-data() -> ()  [unwired: 1 in, 1 out]
        n138 = call "GetSetConfigClass.vi"() -> ("Ref out"=w265:refnum<class "Config.lvclass">)  [unwired: 11 in]
        n139 = property class="Config.lvclass"(reference=w265) -> ("Accessors:PARTF Root Directory"=w264:T42)  [unwired: 1 in, 2 out]
        n140 = Unbundle By Name(w264) -> ("pathRootDir"=w263:path, "ScriptDir"=w262:string)
        n141 = Build Path(base path=w263, name or relative path=w262) -> (appended path=w250:path)
        n142 = call "File Dialog"("start path"=w250, "prompt"="Choose a Monte Carlo Script", "button label"="Script", "pattern (all files)"=w259, "pattern label"=w259) -> ("selected path"=w256:path, "cancelled"=w258:bool, "error out"=w257:errorcluster)  [unwired: 7 in, 1 out]
        n143 = case shown="False" w258 {
          tunnel: w257 -> [w269 w273]
          tunnel: w256 -> [w270 _]
          tunnel: [w272 w273] -> w251
          tunnel: w250 -> [w271 _]
          frame False {
            n144 = call <vilib>:"Compare Two Paths.vi"("error in (no error)"=w269, "Path 2"=w270, "Path 1"=w271) -> ("error out"=w268:errorcluster, "Relative Path from 1 to 2"=w266:path)  [unwired: 5 in, 2 out]
            n145 = Path To String(path=w266) -> (string=w267:string)
            n146 = property on="Monte Carlo Script" class="Str"(error in=w268, "Value"=w267) -> (error out=w272:errorcluster)  [unwired: 1 in, 1 out]
          }
          frame True {
          }
        }
        n147 = call <userlib>:"AddError.vi"("Severity"="Inform", "Priority"=u8 5, "ErrorArray"=w252, "error in (no error)"=w251) -> ("ErrorArray"=w255:errorcluster[])  [unwired: 6 in, 1 out]
      }
      event "btnTestPath": Value Change {
        w283 = "*.tst" ("pattern (all files)")
        n148 = event-data() -> ()  [unwired: 1 in, 1 out]
        n149 = call "GetSetConfigClass.vi"() -> ("Ref out"=w289:refnum<class "Config.lvclass">)  [unwired: 11 in]
        n150 = property class="Config.lvclass"(reference=w289) -> ("Accessors:PARTF Root Directory"=w288:T42)  [unwired: 1 in, 2 out]
        n151 = Unbundle By Name(w288) -> ("pathRootDir"=w287:path, "TestDir"=w286:string)
        n152 = Build Path(base path=w287, name or relative path=w286) -> (appended path=w274:path)
        n153 = call "File Dialog2"("start path"=w274, "prompt"="Choose a Test File", "button label"="Test File", "pattern (all files)"=w283, "pattern label"=w283) -> ("selected path"=w280:path, "cancelled"=w282:bool, "error out"=w281:errorcluster)  [unwired: 7 in, 1 out]
        n154 = case shown="False" w282 {
          tunnel: w281 -> [w294 w297]
          tunnel: w280 -> [w295 _]
          tunnel: [w291 w297] -> w275
          tunnel: w274 -> [w296 _]
          frame False {
            n155 = call <vilib>:"Compare Two Paths.vi"("error in (no error)"=w294, "Path 2"=w295, "Path 1"=w296) -> ("error out"=w292:errorcluster, "Relative Path from 1 to 2"=w293:path)  [unwired: 5 in, 2 out]
            n156 = Path To String(path=w293) -> (string=w290:string)
            n157 = property on="Test File" class="Str"(error in=w292, "Value"=w290) -> (error out=w291:errorcluster)  [unwired: 1 in, 1 out]
          }
          frame True {
          }
        }
        n158 = call <userlib>:"AddError.vi"("Severity"="Inform", "Priority"=u8 5, "ErrorArray"=w276, "error in (no error)"=w275) -> ("ErrorArray"=w279:errorcluster[])  [unwired: 6 in, 1 out]
      }
      event "btnAppConfig": Value Change {
        n159 = event-data() -> ()  [unwired: 1 in, 1 out]
        n160 = call "GetSetFrameworkData.vi"() -> ("clFrameworkData Out"=w303:T30)  [unwired: 11 in]
        n161 = Unbundle By Name(w303) -> ("AppModuleID"=w302:i32)
        n162 = call "OpenAppConfigRequest.vi"("ModuleID"=w302) -> ("error out"=w300:errorcluster)  [unwired: 10 in]
        n163 = call <userlib>:"AddError.vi"("Severity"="Abort", "Priority"=u8 3, "error in (no error)"=w300) -> ("ErrorArray"=w301:errorcluster[])  [unwired: 7 in, 1 out]
      }
      event "btnVisualize": Value Change {
        n164 = event-data() -> ()  [unwired: 1 in, 1 out]
        n165 = call "Enqueue.vi"("ErrorArray"=w305, "Msg"="Visualize") -> ("ErrorArray"=w304:errorcluster[])  [unwired: 9 in]
      }
      event "Number of Buses": Value Change {
        w310 = T43."Disabled and Grayed Out" ("Action")
        w311 = T43."Enabled" ("Action")
        # "No active buses."
        n166 = event-data() -> ("NewVal"=w316:u8)  [unwired: 1 in]
        n167 = call "GetButtonRefs.vi"() -> ("BtnRefs"=w307:T4)  [unwired: 11 in]
        n168 = Greater Than 0?(x=w316) -> (x > 0?=w312:bool)
        n169 = Select(t=w311, s=w312, f=w310) -> (s? t:f=w313:T43)
        n170 = Select(t=w310, s=w312, f=w311) -> (s? t:f=w308:T43)
        n171 = Unbundle By Name(w307) -> ("AppTypeRef"=w309:refnum<vi>)
        n172 = property class="Ring (strict)"(reference=w309, "DisabledEnum"=w308) -> ()  [unwired: 1 in, 2 out]
        n173 = call "EnableDisableButtons.vi"("Action"=w313, "ErrorArray In"=w315) -> ("ErrorArray Out"=w314:errorcluster[])  [unwired: 9 in]
      }
      event "Bus Number": Value Change {
        n174 = event-data() -> ()  [unwired: 1 in, 1 out]
        n175 = call "Enqueue.vi"("Priority (f)"=TRUE, "ErrorArray"=w318, "Msg"="UpdateFrontPanel") -> ("ErrorArray"=w317:errorcluster[])  [unwired: 8 in]
      }
      event "Event Type": Value Change {
        # "If the value of Event Type is changed, update Event Params\nto defaults with appropriate row and column headers."
        n176 = event-data() -> ()  [unwired: 1 in, 1 out]
        n177 = call "InitEvtParams.vi"("ErrorArray In"=w322) -> ("ErrorArray Out"=w321:errorcluster[])  [unwired: 10 in]
      }
      event "Sensor Impairment Type": Value Change {
        # "If the value of PMU Impairment Type is changed, \nupdate PMU Impairment Params to defaults with\nappropriate row and column headers."
        n178 = event-data() -> ()  [unwired: 1 in, 1 out]
        n179 = call "InitPmuImpairParams.vi"("ErrorArray In"=w324) -> ("ErrorArray Out"=w323:errorcluster[])  [unwired: 10 in]
      }
      event "Status Impairment Type": Value Change {
        n180 = event-data() -> ()  [unwired: 1 in, 2 out]
        n181 = call "InitFlagImpairParams.vi"("ErrorArray In"=w326) -> ("ErrorArray Out"=w325:errorcluster[])  [unwired: 10 in]
      }
      event "Network Impairment Type": Value Change {
        n182 = event-data() -> ()  [unwired: 1 in, 2 out]
        n183 = call "InitNetworkImpairParams.vi"("ErrorArray In"=w328) -> ("ErrorArray Out"=w327:errorcluster[])  [unwired: 10 in]
      }
      event "Event Parameters": Value Change {
        # "If EvtParams are changed, check to make sure that\nthe input is a number.  If it is not, don't accept the change\nand revert table to last acceptable value."
        n184 = event-data() -> ("NewVal"=w333:string[][], "OldVal"=w332:string[][])  [unwired: 1 in]
        n185 = control-ref of="Event Parameters"() -> (w329:refnum<vi>)
        n186 = call "CheckTableIsNumeric.vi"("ErrorArray In"=w331, "strOldVal"=w332, "strNewVal"=w333, "TableRefnum"=w329) -> ("ErrorArray Out"=w330:errorcluster[])  [unwired: 7 in]
      }
      event Value Change {
        # "Event Config PosSeq and PMU Impair Config PosSeq should always match"
        n187 = event-data() -> ("NewVal"=w338:bool)  [unwired: 1 in]
        n188 = call "GetControlRefs.vi"() -> ("clControlRefs Out"=w335:T5)  [unwired: 11 in]
        n189 = Unbundle By Name(w335) -> ("PmuImpairConfigRef"=w334:refnum<vi>)
        n190 = property class="Clust (strict)"(reference=w334) -> (reference out=w337:refnum<vi>, "Value"=w339:T2)  [unwired: 1 in, 1 out]
        n191 = Bundle By Name(cluster=w339, "bPosSeq"=w338) -> (w336:T2)
        n192 = property class="Clust (strict)"(reference=w337, "Value"=w336) -> ()  [unwired: 1 in, 2 out]
      }
      event Value Change {
        # "Event Config PosSeq and PMU Impair Config PosSeq should always match"
        n193 = event-data() -> ("NewVal"=w344:bool)  [unwired: 1 in]
        n194 = call "GetControlRefs.vi"() -> ("clControlRefs Out"=w341:T5)  [unwired: 11 in]
        n195 = Unbundle By Name(w341) -> ("EvtConfigRef"=w340:refnum<vi>)
        n196 = property class="Clust (strict)"(reference=w340) -> (reference out=w343:refnum<vi>, "Value"=w345:T3)  [unwired: 1 in, 1 out]
        n197 = Bundle By Name(cluster=w345, "PosSeq"=w344) -> (w342:T3)
        n198 = property class="Clust (strict)"(reference=w343, "Value"=w342) -> ()  [unwired: 1 in, 2 out]
      }
      event "Sensor Impairment Parameters": Value Change {
        # "If PmuImpairParams are changed, check to make sure that\nthe input is a number.  If it is not, don't accept the change\nand revert table to last acceptable value."
        n199 = event-data() -> ("NewVal"=w347:string[][], "OldVal"=w348:string[][])  [unwired: 1 in]
        n200 = control-ref of="Sensor Impairment Parameters"() -> (w346:refnum<vi>)
        n201 = call "CheckTableIsNumeric.vi"("ErrorArray In"=w350, "strOldVal"=w348, "strNewVal"=w347, "TableRefnum"=w346) -> ("ErrorArray Out"=w349:errorcluster[])  [unwired: 7 in]
      }
      event "Network Impairment Parameters": Value Change {
        # "If NetworkImpairParams are changed, check to make sure that\nthe input is a number.  If it is not, don't accept the change\nand revert table to last acceptable value."
        n202 = event-data() -> ("NewVal"=w353:string[][], "OldVal"=w354:string[][])  [unwired: 1 in]
        n203 = control-ref of="Network Impairment Parameters"() -> (w352:refnum<vi>)
        n204 = call "CheckTableIsNumeric.vi"("ErrorArray In"=w355, "strOldVal"=w354, "strNewVal"=w353, "TableRefnum"=w352) -> ("ErrorArray Out"=w351:errorcluster[])  [unwired: 7 in]
      }
      event "Status Impairment Parameters": Value Change {
        # "If FlagImpairParams are changed, check to make sure that\nthe input is a number.  If it is not, don't accept the change\nand revert table to last acceptable value."
        n205 = event-data() -> ("NewVal"=w358:string[][], "OldVal"=w359:string[][])  [unwired: 1 in]
        n206 = control-ref of="Status Impairment Parameters"() -> (w357:refnum<vi>)
        n207 = call "CheckTableIsNumeric.vi"("ErrorArray In"=w360, "strOldVal"=w359, "strNewVal"=w358, "TableRefnum"=w357) -> ("ErrorArray Out"=w356:errorcluster[])  [unwired: 7 in]
      }
      event Value Change {
        # "If the Nominal Frequency is changed, populate the \nReporting Rate with the appropriate array of values."
        n208 = event-data() -> ("NewVal"=w361:u16)  [unwired: 1 in]
        n209 = call "PopReportingRate.vi"("ErrorArray In"=w363, "Nominal Frequency (60)"=w361) -> ("ErrorArray Out"=w362:errorcluster[])  [unwired: 9 in]
      }
      event User Event {
        n210 = event-data() -> ()  [unwired: 1 in, 1 out]
        n211 = call "Enqueue.vi"("Priority (f)"=TRUE, "ErrorArray"=w366, "Msg"="Stop") -> ("ErrorArray"=w365:errorcluster[])  [unwired: 8 in]
      }
      event User Event {
        n212 = event-data() -> ("Data"=w372:variant)  [unwired: 1 in]
        n213 = Variant To Data(type=T13 {"Init?"=FALSE, "ModuleAdmin"=refnum} ("clDidInit"), Variant=w372) -> (data=w383:T13, error out=w382:errorcluster)  [unwired: 1 in]
        n214 = Unbundle By Name(w383) -> ("ModuleAdmin"=w377:refnum<class "ModuleAdmin.lvclass">)
        n215 = Get Date/Time In Seconds() -> (seconds since 1Jan1904=w387:timestamp)
        n216 = property class="ModuleAdmin.lvclass"(reference=w377) -> ("Accessors:ModuleName"=w376:string, "Accessors:Module ID"=w375:i32)  [unwired: 1 in, 2 out]
        n217 = Get Date/Time String(date format (0)=enum16{"short", "long", "abbreviated"}."short", seconds (now)=w387, want seconds? (F)=TRUE) -> (time string=w389:string)  [unwired: 1 out]
        n218 = Format Into String(format string="%s: %s: %d %s \\r", error in=w382, w389, w376, w375, "Did Init.") -> (resulting string=w370:string, error out=w371:errorcluster)  [unwired: 1 in]
        n219 = call "AddLogMsg.vi"("error in (no error)"=w371, "LogMessage"=w370) -> ("error out"=w369:errorcluster)  [unwired: 9 in]
        n220 = call <userlib>:"AddError.vi"("Severity"="Inform" ("String"), "Priority"=u8 4, "ErrorArray"=w374, "error in (no error)"=w369) -> ("ErrorArray"=w373:errorcluster[], "error out"=w379:errorcluster)  [unwired: 6 in]
        n221 = call <vilib>:"Clear Errors.vi"("error in (no error)"=w379) -> ()  [unwired: 5 in, 2 out]
      }
      event User Event {
        n222 = event-data() -> ("Data"=w394:variant)  [unwired: 1 in]
        n223 = Variant To Data(type=T14 {"Status"=""} ("clStatUpdate"), Variant=w394) -> (data=w406:T14, error out=w399:errorcluster)  [unwired: 1 in]
        n224 = Unbundle By Name(w406) -> ("Status"=w400:string)
        n225 = Get Date/Time In Seconds() -> (seconds since 1Jan1904=w404:timestamp)
        n226 = Get Date/Time String(date format (0)=enum16{"short", "long", "abbreviated"}."short", seconds (now)=w404, want seconds? (F)=TRUE) -> (time string=w401:string)  [unwired: 1 out]
        n227 = Format Into String(format string="%s: %s \\r", error in=w399, w401, w400) -> (resulting string=w391:string, error out=w392:errorcluster)  [unwired: 1 in]
        n228 = call "AddLogMsg.vi"("error in (no error)"=w392, "LogMessage"=w391) -> ("error out"=w390:errorcluster)  [unwired: 9 in]
        n229 = call <userlib>:"AddError.vi"("Severity"="Inform" ("String"), "Priority"=u8 4, "ErrorArray"=w395, "error in (no error)"=w390) -> ("ErrorArray"=w393:errorcluster[], "error out"=w396:errorcluster)  [unwired: 6 in]
        n230 = call <vilib>:"Clear Errors.vi"("error in (no error)"=w396) -> ()  [unwired: 5 in, 2 out]
      }
      event User Event {
        n231 = event-data() -> ("Data"=w408:variant)  [unwired: 1 in]
        n232 = Variant To Data(type=T15 {"error"={"status"=FALSE, "code"=0, "source"=""}, "AdditionalInfo"=""} ("Cluster"), Variant=w408) -> (data=w415:T15)  [unwired: 1 in, 1 out]
        n233 = Unbundle By Name(w415) -> ("error"=w411:errorcluster)
        n234 = call <userlib>:"AddError.vi"("Severity"="UserOption" ("String"), "Priority"=u8 2, "ErrorArray"=w409, "error in (no error)"=w411) -> ("ErrorArray"=w410:errorcluster[], "error out"=w412:errorcluster)  [unwired: 6 in]
        n235 = call <vilib>:"Clear Errors.vi"("error in (no error)"=w412) -> ()  [unwired: 5 in, 2 out]
      }
      event User Event {
        n236 = event-data() -> ("Data"=w421:variant)  [unwired: 1 in]
        n237 = Get Date/Time In Seconds() -> (seconds since 1Jan1904=w435:timestamp)
        n238 = Get Date/Time String(date format (0)=enum16{"short", "long", "abbreviated"}."short", seconds (now)=w435, want seconds? (F)=TRUE) -> (time string=w437:string)  [unwired: 1 out]
        n239 = Variant To Data(type=T16 {"Exit via Stop Module Req?"=FALSE, "Wait for Module to stop?"=FALSE, "ModuleAdmin"=refnum} ("Stop Argument"), Variant=w421) -> (data=w432:T16, error out=w430:errorcluster)  [unwired: 1 in]
        n240 = Unbundle By Name(w432) -> ("ModuleAdmin"=w425:refnum<class "ModuleAdmin.lvclass">)
        n241 = property class="ModuleAdmin.lvclass"(reference=w425) -> ("Accessors:ModuleName"=w424:string, "Accessors:Module ID"=w423:i32)  [unwired: 1 in, 2 out]
        n242 = Format Into String(format string="%s: %s: %d %s \\r", error in=w430, w437, w424, w423, "Stopping") -> (resulting string=w418:string, error out=w419:errorcluster)  [unwired: 1 in]
        n243 = call "AddLogMsg.vi"("error in (no error)"=w419, "LogMessage"=w418) -> ("error out"=w417:errorcluster)  [unwired: 9 in]
        n244 = call <userlib>:"AddError.vi"("Severity"="Inform" ("String"), "Priority"=u8 4, "ErrorArray"=w420, "error in (no error)"=w417) -> ("ErrorArray"=w422:errorcluster[], "error out"=w427:errorcluster)  [unwired: 6 in]
        n245 = call <vilib>:"Clear Errors.vi"("error in (no error)"=w427) -> ()  [unwired: 5 in, 2 out]
      }
      event User Event {
        n246 = event-data() -> ("Data"=w441:variant)  [unwired: 1 in]
        n247 = Variant To Data(type=T17 {"Init?"=FALSE, "ModuleAdmin"=refnum} ("clDidInit"), Variant=w441) -> (data=w452:T17, error out=w451:errorcluster)  [unwired: 1 in]
        n248 = Unbundle By Name(w452) -> ("ModuleAdmin"=w446:refnum<class "ModuleAdmin.lvclass">)
        n249 = Get Date/Time In Seconds() -> (seconds since 1Jan1904=w456:timestamp)
        n250 = Get Date/Time String(date format (0)=enum16{"short", "long", "abbreviated"}."short", seconds (now)=w456, want seconds? (F)=TRUE) -> (time string=w458:string)  [unwired: 1 out]
        n251 = property class="ModuleAdmin.lvclass"(reference=w446) -> ("Accessors:ModuleName"=w445:string, "Accessors:Module ID"=w444:i32)  [unwired: 1 in, 2 out]
        n252 = Format Into String(format string="%s: %s: %d %s \\r", error in=w451, w458, w445, w444, "Did Init.") -> (resulting string=w439:string, error out=w440:errorcluster)  [unwired: 1 in]
        n253 = call "AddLogMsg.vi"("error in (no error)"=w440, "LogMessage"=w439) -> ("error out"=w438:errorcluster)  [unwired: 9 in]
        n254 = call <userlib>:"AddError.vi"("Severity"="Inform" ("String"), "Priority"=u8 4, "ErrorArray"=w443, "error in (no error)"=w438) -> ("ErrorArray"=w442:errorcluster[], "error out"=w448:errorcluster)  [unwired: 6 in]
        n255 = call <vilib>:"Clear Errors.vi"("error in (no error)"=w448) -> ()  [unwired: 5 in, 2 out]
      }
      event User Event {
        n256 = event-data() -> ("Data"=w463:variant)  [unwired: 1 in]
        n257 = Variant To Data(type=T18 {"Status"=""} ("clStatUpdate"), Variant=w463) -> (data=w475:T18, error out=w468:errorcluster)  [unwired: 1 in]
        n258 = Unbundle By Name(w475) -> ("Status"=w469:string)
        n259 = Get Date/Time In Seconds() -> (seconds since 1Jan1904=w473:timestamp)
        n260 = Get Date/Time String(date format (0)=enum16{"short", "long", "abbreviated"}."short", seconds (now)=w473, want seconds? (F)=TRUE) -> (time string=w470:string)  [unwired: 1 out]
        n261 = Format Into String(format string="%s: %s \\r", error in=w468, w470, w469) -> (resulting string=w460:string, error out=w461:errorcluster)  [unwired: 1 in]
        n262 = call "AddLogMsg.vi"("error in (no error)"=w461, "LogMessage"=w460) -> ("error out"=w459:errorcluster)  [unwired: 9 in]
        n263 = call <userlib>:"AddError.vi"("Severity"="Inform" ("String"), "Priority"=u8 4, "ErrorArray"=w462, "error in (no error)"=w459) -> ("ErrorArray"=w464:errorcluster[], "error out"=w465:errorcluster)  [unwired: 6 in]
        n264 = call <vilib>:"Clear Errors.vi"("error in (no error)"=w465) -> ()  [unwired: 5 in, 2 out]
      }
      event User Event {
        n265 = event-data() -> ("Data"=w477:variant)  [unwired: 1 in]
        n266 = Variant To Data(type=T19 {"error"={"status"=FALSE, "code"=0, "source"=""}, "AdditionalInfo"=""} ("Cluster"), Variant=w477) -> (data=w484:T19)  [unwired: 1 in, 1 out]
        n267 = Unbundle By Name(w484) -> ("error"=w480:errorcluster)
        n268 = call <userlib>:"AddError.vi"("Severity"="UserOption" ("String"), "Priority"=u8 2, "ErrorArray"=w478, "error in (no error)"=w480) -> ("ErrorArray"=w479:errorcluster[], "error out"=w481:errorcluster)  [unwired: 6 in]
        n269 = call <vilib>:"Clear Errors.vi"("error in (no error)"=w481) -> ()  [unwired: 5 in, 2 out]
      }
      event User Event {
        n270 = event-data() -> ("Data"=w490:variant)  [unwired: 1 in]
        n271 = Variant To Data(type=T20 {"Exit via Stop Module Req?"=FALSE, "Wait for Module to stop?"=FALSE, "ModuleAdmin"=refnum} ("Stop Argument"), Variant=w490) -> (data=w501:T20, error out=w499:errorcluster)  [unwired: 1 in]
        n272 = Get Date/Time In Seconds() -> (seconds since 1Jan1904=w504:timestamp)
        n273 = Get Date/Time String(date format (0)=enum16{"short", "long", "abbreviated"}."short", seconds (now)=w504, want seconds? (F)=TRUE) -> (time string=w506:string)  [unwired: 1 out]
        n274 = Unbundle By Name(w501) -> ("ModuleAdmin"=w494:refnum<class "ModuleAdmin.lvclass">)
        n275 = property class="ModuleAdmin.lvclass"(reference=w494) -> ("Accessors:ModuleName"=w493:string, "Accessors:Module ID"=w492:i32)  [unwired: 1 in, 2 out]
        n276 = Format Into String(format string="%s: %s: %d %s \\r", error in=w499, w506, w493, w492, "Stopping") -> (resulting string=w487:string, error out=w488:errorcluster)  [unwired: 1 in]
        n277 = call "AddLogMsg.vi"("error in (no error)"=w488, "LogMessage"=w487) -> ("error out"=w486:errorcluster)  [unwired: 9 in]
        n278 = call <userlib>:"AddError.vi"("Severity"="Inform" ("String"), "Priority"=u8 4, "ErrorArray"=w489, "error in (no error)"=w486) -> ("ErrorArray"=w491:errorcluster[], "error out"=w496:errorcluster)  [unwired: 6 in]
        n279 = call <vilib>:"Clear Errors.vi"("error in (no error)"=w496) -> ()  [unwired: 5 in, 2 out]
      }
      event User Event {
        n280 = event-data() -> ("Data"=w508:variant)  [unwired: 1 in]
        n281 = Variant To Data(type=T21 {"Init?"=FALSE, "ModuleAdmin"=refnum} ("clDidInit"), Variant=w508) -> (data=w521:T21, error out=w520:errorcluster)  [unwired: 1 in]
        n282 = Unbundle By Name(w521) -> ("ModuleAdmin"=w515:refnum<class "ModuleAdmin.lvclass">)
        n283 = Get Date/Time In Seconds() -> (seconds since 1Jan1904=w525:timestamp)
        n284 = Get Date/Time String(date format (0)=enum16{"short", "long", "abbreviated"}."short", seconds (now)=w525, want seconds? (F)=TRUE) -> (time string=w527:string)  [unwired: 1 out]
        n285 = property class="ModuleAdmin.lvclass"(reference=w515) -> ("Accessors:ModuleName"=w514:string, "Accessors:Module ID"=w513:i32)  [unwired: 1 in, 2 out]
        n286 = Format Into String(format string="%s: %s: %d %s \\r", error in=w520, w527, w514, w513, "Did Init.") -> (resulting string=w511:string, error out=w512:errorcluster)  [unwired: 1 in]
        n287 = call "AddLogMsg.vi"("error in (no error)"=w512, "LogMessage"=w511) -> ("error out"=w510:errorcluster)  [unwired: 9 in]
        n288 = call <userlib>:"AddError.vi"("Severity"="Inform" ("String"), "Priority"=u8 4, "ErrorArray"=w509, "error in (no error)"=w510) -> ("ErrorArray"=w507:errorcluster[], "error out"=w517:errorcluster)  [unwired: 6 in]
        n289 = call <vilib>:"Clear Errors.vi"("error in (no error)"=w517) -> ()  [unwired: 5 in, 2 out]
      }
      event User Event {
        n290 = event-data() -> ("Data"=w531:variant)  [unwired: 1 in]
        n291 = Variant To Data(type=T22 {"Status"=""} ("clStatUpdate"), Variant=w531) -> (data=w544:T22, error out=w538:errorcluster)  [unwired: 1 in]
        n292 = Unbundle By Name(w544) -> ("Status"=w539:string)
        n293 = Get Date/Time In Seconds() -> (seconds since 1Jan1904=w543:timestamp)
        n294 = Get Date/Time String(date format (0)=enum16{"short", "long", "abbreviated"}."short", seconds (now)=w543, want seconds? (F)=TRUE) -> (time string=w540:string)  [unwired: 1 out]
        n295 = Format Into String(format string="%s: %s \\r", error in=w538, w540, w539) -> (resulting string=w533:string, error out=w534:errorcluster)  [unwired: 1 in]
        n296 = call "AddLogMsg.vi"("error in (no error)"=w534, "LogMessage"=w533) -> ("error out"=w532:errorcluster)  [unwired: 9 in]
        n297 = call <userlib>:"AddError.vi"("Severity"="Inform" ("String"), "Priority"=u8 4, "ErrorArray"=w530, "error in (no error)"=w532) -> ("ErrorArray"=w529:errorcluster[], "error out"=w535:errorcluster)  [unwired: 6 in]
        n298 = call <vilib>:"Clear Errors.vi"("error in (no error)"=w535) -> ()  [unwired: 5 in, 2 out]
      }
      event User Event {
        n299 = event-data() -> ("Data"=w547:variant)  [unwired: 1 in]
        n300 = Variant To Data(type=T23 {"error"={"status"=FALSE, "code"=0, "source"=""}, "AdditionalInfo"=""} ("Cluster"), Variant=w547) -> (data=w553:T23)  [unwired: 1 in, 1 out]
        n301 = Unbundle By Name(w553) -> ("error"=w549:errorcluster)
        n302 = call <userlib>:"AddError.vi"("Severity"="UserOption" ("String"), "Priority"=u8 2, "ErrorArray"=w548, "error in (no error)"=w549) -> ("ErrorArray"=w546:errorcluster[], "error out"=w550:errorcluster)  [unwired: 6 in]
        n303 = call <vilib>:"Clear Errors.vi"("error in (no error)"=w550) -> ()  [unwired: 5 in, 2 out]
      }
      event User Event {
        n304 = event-data() -> ("Data"=w555:variant)  [unwired: 1 in]
        n305 = Variant To Data(type=T24 {"Exit via Stop Module Req?"=FALSE, "Wait for Module to stop?"=FALSE, "ModuleAdmin"=refnum} ("Stop Argument"), Variant=w555) -> (data=w570:T24, error out=w568:errorcluster)  [unwired: 1 in]
        n306 = Get Date/Time In Seconds() -> (seconds since 1Jan1904=w573:timestamp)
        n307 = Get Date/Time String(date format (0)=enum16{"short", "long", "abbreviated"}."short", seconds (now)=w573, want seconds? (F)=TRUE) -> (time string=w575:string)  [unwired: 1 out]
        n308 = Unbundle By Name(w570) -> ("ModuleAdmin"=w563:refnum<class "ModuleAdmin.lvclass">)
        n309 = property class="ModuleAdmin.lvclass"(reference=w563) -> ("Accessors:ModuleName"=w562:string, "Accessors:Module ID"=w561:i32)  [unwired: 1 in, 2 out]
        n310 = Format Into String(format string="%s: %s: %d %s \\r", error in=w568, w575, w562, w561, "Stopping") -> (resulting string=w559:string, error out=w560:errorcluster)  [unwired: 1 in]
        n311 = call "AddLogMsg.vi"("error in (no error)"=w560, "LogMessage"=w559) -> ("error out"=w558:errorcluster)  [unwired: 9 in]
        n312 = call <userlib>:"AddError.vi"("Severity"="Inform" ("String"), "Priority"=u8 4, "ErrorArray"=w556, "error in (no error)"=w558) -> ("ErrorArray"=w557:errorcluster[], "error out"=w565:errorcluster)  [unwired: 6 in]
        n313 = call <vilib>:"Clear Errors.vi"("error in (no error)"=w565) -> ()  [unwired: 5 in, 2 out]
      }
      event User Event {
        n314 = event-data() -> ("Data"=w578:variant)  [unwired: 1 in]
        n315 = Variant To Data(type=T25 {"Init?"=FALSE, "ModuleAdmin"=refnum} ("clDidInit"), Variant=w578) -> (data=w590:T25, error out=w589:errorcluster)  [unwired: 1 in]
        n316 = Unbundle By Name(w590) -> ("ModuleAdmin"=w584:refnum<class "ModuleAdmin.lvclass">)
        n317 = Get Date/Time In Seconds() -> (seconds since 1Jan1904=w594:timestamp)
        n318 = Get Date/Time String(date format (0)=enum16{"short", "long", "abbreviated"}."short", seconds (now)=w594, want seconds? (F)=TRUE) -> (time string=w596:string)  [unwired: 1 out]
        n319 = property class="ModuleAdmin.lvclass"(reference=w584) -> ("Accessors:ModuleName"=w583:string, "Accessors:Module ID"=w582:i32)  [unwired: 1 in, 2 out]
        n320 = Format Into String(format string="%s: %s: %d %s \\r", error in=w589, w596, w583, w582, "Did Init.") -> (resulting string=w580:string, error out=w581:errorcluster)  [unwired: 1 in]
        n321 = call "AddLogMsg.vi"("error in (no error)"=w581, "LogMessage"=w580) -> ("error out"=w579:errorcluster)  [unwired: 9 in]
        n322 = call <userlib>:"AddError.vi"("Severity"="Inform" ("String"), "Priority"=u8 4, "ErrorArray"=w577, "error in (no error)"=w579) -> ("ErrorArray"=w576:errorcluster[], "error out"=w586:errorcluster)  [unwired: 6 in]
        n323 = call <vilib>:"Clear Errors.vi"("error in (no error)"=w586) -> ()  [unwired: 5 in, 2 out]
      }
      event User Event {
        n324 = event-data() -> ("Data"=w598:variant)  [unwired: 1 in]
        n325 = Variant To Data(type=T26 {"Status"=""} ("clStatUpdate"), Variant=w598) -> (data=w613:T26, error out=w607:errorcluster)  [unwired: 1 in]
        n326 = Unbundle By Name(w613) -> ("Status"=w608:string)
        n327 = Get Date/Time In Seconds() -> (seconds since 1Jan1904=w612:timestamp)
        n328 = Get Date/Time String(date format (0)=enum16{"short", "long", "abbreviated"}."short", seconds (now)=w612, want seconds? (F)=TRUE) -> (time string=w609:string)  [unwired: 1 out]
        n329 = Format Into String(format string="%s: %s \\r", error in=w607, w609, w608) -> (resulting string=w602:string, error out=w603:errorcluster)  [unwired: 1 in]
        n330 = call "AddLogMsg.vi"("error in (no error)"=w603, "LogMessage"=w602) -> ("error out"=w601:errorcluster)  [unwired: 9 in]
        n331 = call <userlib>:"AddError.vi"("Severity"="Inform" ("String"), "Priority"=u8 4, "ErrorArray"=w597, "error in (no error)"=w601) -> ("ErrorArray"=w599:errorcluster[], "error out"=w604:errorcluster)  [unwired: 6 in]
        n332 = call <vilib>:"Clear Errors.vi"("error in (no error)"=w604) -> ()  [unwired: 5 in, 2 out]
      }
      event User Event {
        n333 = event-data() -> ("Data"=w616:variant)  [unwired: 1 in]
        n334 = Variant To Data(type=T27 {"error"={"status"=FALSE, "code"=0, "source"=""}, "AdditionalInfo"=""} ("Cluster"), Variant=w616) -> (data=w622:T27)  [unwired: 1 in, 1 out]
        n335 = Unbundle By Name(w622) -> ("error"=w618:errorcluster)
        n336 = call <userlib>:"AddError.vi"("Severity"="UserOption" ("String"), "Priority"=u8 2, "ErrorArray"=w615, "error in (no error)"=w618) -> ("ErrorArray"=w617:errorcluster[], "error out"=w619:errorcluster)  [unwired: 6 in]
        n337 = call <vilib>:"Clear Errors.vi"("error in (no error)"=w619) -> ()  [unwired: 5 in, 2 out]
      }
      event User Event {
        n338 = event-data() -> ("Data"=w624:variant)  [unwired: 1 in]
        n339 = Variant To Data(type=T28 {"Exit via Stop Module Req?"=FALSE, "Wait for Module to stop?"=FALSE, "ModuleAdmin"=refnum} ("Stop Argument"), Variant=w624) -> (data=w639:T28, error out=w637:errorcluster)  [unwired: 1 in]
        n340 = Get Date/Time In Seconds() -> (seconds since 1Jan1904=w642:timestamp)
        n341 = Get Date/Time String(date format (0)=enum16{"short", "long", "abbreviated"}."short", seconds (now)=w642, want seconds? (F)=TRUE) -> (time string=w644:string)  [unwired: 1 out]
        n342 = Unbundle By Name(w639) -> ("ModuleAdmin"=w632:refnum<class "ModuleAdmin.lvclass">)
        n343 = property class="ModuleAdmin.lvclass"(reference=w632) -> ("Accessors:ModuleName"=w631:string, "Accessors:Module ID"=w630:i32)  [unwired: 1 in, 2 out]
        n344 = Format Into String(format string="%s: %s: %d %s \\r", error in=w637, w644, w631, w630, "Stopping") -> (resulting string=w628:string, error out=w629:errorcluster)  [unwired: 1 in]
        n345 = call "AddLogMsg.vi"("error in (no error)"=w629, "LogMessage"=w628) -> ("error out"=w627:errorcluster)  [unwired: 9 in]
        n346 = call <userlib>:"AddError.vi"("Severity"="Inform" ("String"), "Priority"=u8 4, "ErrorArray"=w625, "error in (no error)"=w627) -> ("ErrorArray"=w626:errorcluster[], "error out"=w634:errorcluster)  [unwired: 6 in]
        n347 = call <vilib>:"Clear Errors.vi"("error in (no error)"=w634) -> ()  [unwired: 5 in, 2 out]
      }
      event User Event {
        n348 = event-data() -> ("Data"=w647:variant)  [unwired: 1 in]
        n349 = Variant To Data(type=T29 {"error"={"status"=FALSE, "code"=0, "source"=""}, "AdditionalInfo"=""} ("Cluster"), Variant=w647) -> (data=w653:T29)  [unwired: 1 in, 1 out]
        n350 = Unbundle By Name(w653) -> ("error"=w649:errorcluster)
        n351 = call <userlib>:"AddError.vi"("Severity"="UserOption" ("String"), "Priority"=u8 2, "ErrorArray"=w646, "error in (no error)"=w649) -> ("ErrorArray"=w648:errorcluster[], "error out"=w650:errorcluster)  [unwired: 6 in]
        n352 = call <vilib>:"Clear Errors.vi"("error in (no error)"=w650) -> ()  [unwired: 5 in, 2 out]
      }
    }
    n353 = call "EnqueueError.vi"("ErrorArray"=w68) -> ("ErrorArray"=w67:errorcluster[])  [unwired: 10 in]
  }
  n354 = while {
    shift-right: [w655] -> _
    shift-left: w61 -> [w659]
    stop <- w660 stop-if-true
    # "Queued Message Handler"
    n355 = call "Dequeue.vi"("ErrorArray"=w659) -> ("ErrorArray"=w656:errorcluster[], "Data"=w657:variant, "Msg"=w658:string)  [unwired: 8 in]
    n356 = case shown="\"Visualize\"" w658 {
      selector: w658 -> [w667 _ _ _ _ _ _ _ _ _ _ _ _ _ _]
      tunnel: [_ _ _ _ _ _ _ _ _ _ _ _ _ _ w833] -> w660
      tunnel: w657 -> [_ _ _ _ _ w712 w716 _ _ _ _ _ w784 w800 _]
      tunnel: w656 -> [w664 w676 w697 w701 w703 w710 w717 w722 w750 w772 w780 w781 w785 _ w834]
      tunnel: [w662 w675 w684 w698 w702 w704 w714 w718 w752 w768 w779 w782 w783 w794 w829] -> w654
      frame Default {
        n357 = xnode "Error Ring"("parameter 0"=w667) -> ("error out"=w666:errorcluster)
        n358 = call <userlib>:"AddError.vi"("Severity"="Inform" ("String"), "Priority"=u8 5, "ErrorArray"=w664, "error in (no error)"=w666) -> ("ErrorArray"=w662:errorcluster[], "error out"=w661:errorcluster)  [unwired: 6 in]
        n359 = call <vilib>:"Clear Errors.vi"("error in (no error)"=w661) -> ()  [unwired: 5 in, 2 out]
      }
      frame "Initialize" {
        n360 = call "InitFrontPanel.vi"("ErrorArray In"=w676) -> ("ErrorArray Out"=w675:errorcluster[])  [unwired: 10 in]
      }
      frame "UpdateBusFromFrontPanel" {
        # "Update the data in each module within the selected bus from the front panel control values."
        n361 = call "UpdateBusFromFrontPanel.vi"("ErrorArray In"=w697) -> ("ErrorArray Out"=w696:errorcluster[], "output cluster"=w695:T32, "Framework.lvlib:Bus.lvclass"=w694:refnum<class "Bus.lvclass">)  [unwired: 8 in]
        n362 = call "UpdateEvent.vi"("ErrorArray In"=w696, "clBusData In"=w695, "Bus.lvclass In"=w694) -> ("ErrorArray Out"=w693:errorcluster[], "clBusData Out"=w692:T32, "Bus.lvclass Out"=w691:refnum<class "Bus.lvclass">)  [unwired: 6 in]
        n363 = call "UpdatePmuImpairment.vi"("ErrorArray In"=w693, "clBusData In"=w692, "Bus.lvclass In"=w691) -> ("ErrorArray Out"=w690:errorcluster[], "clBusData Out"=w689:T32, "Bus.lvclass Out"=w688:refnum<class "Bus.lvclass">)  [unwired: 6 in]
        n364 = call "UpdateNetworkImpairment.vi"("ErrorArray In"=w690, "clBusData In"=w689, "Bus.lvclass In"=w688) -> ("ErrorArray Out"=w687:errorcluster[], "clBusData Out"=w686:T32, "Bus.lvclass Out"=w685:refnum<class "Bus.lvclass">)  [unwired: 6 in]
        n365 = call "UpdateFlagImpairment.vi"("ErrorArray In"=w687, "clBusData In"=w686, "Bus.lvclass In"=w685) -> ("ErrorArray Out"=w683:errorcluster[], "clBusData Out"=w681:T32, "Bus.lvclass Out"=w680:refnum<class "Bus.lvclass">)  [unwired: 6 in]
        n366 = call "UpdateApp.vi"("DefaultAppConfig? (f)"=FALSE, "ErrorArray In"=w683, "clBusData in"=w681, "Bus.lvclass"=w680) -> ("ErrorArray Out"=w682:errorcluster[], "clBusData out"=w678:T32, "Bus.lvclass"=w679:refnum<class "Bus.lvclass">)  [unwired: 5 in]
        n367 = call "UpdateOutputToFile.vi"("ErrorArray In"=w682, "clBusData In"=w678, "Bus.lvclass In"=w679) -> ("ErrorArray Out"=w684:errorcluster[])  [unwired: 6 in, 2 out]
      }
      frame "RemoveBus" {
        # "ditto"
        # "Remove the App when the last bus is removed"
        # "Remove bus selected on front panel."
        n368 = call "RemoveBus.vi"("ErrorArray In"=w701) -> ("ErrorArray Out"=w700:errorcluster[])  [unwired: 10 in]
        n369 = call "RemoveApp.vi"("ErrorArray In"=w700) -> ("ErrorArray Out"=w699:errorcluster[])  [unwired: 10 in]
        n370 = call "RemoveOutToFile.vi"("ErrorArray In"=w699) -> ("ErrorArray Out"=w698:errorcluster[])  [unwired: 10 in]
      }
      frame "UpdateFrontPanel" {
        n371 = call "UpdateFrontPanel.vi"("ErrorArray In"=w703) -> ("ErrorArray Out"=w702:errorcluster[])  [unwired: 10 in]
      }
      frame "get" {
        n372 = Variant To Data(type="", Variant=w712) -> (data=w705:string, error out=w706:errorcluster)  [unwired: 1 in]
        n373 = call <userlib>:"AddError.vi"("Severity"="Abort", "Priority"=u8 3, "ErrorArray"=w710, "error in (no error)"=w706) -> ("ErrorArray"=w707:errorcluster[])  [unwired: 6 in, 1 out]
        n374 = call "LtaGet.vi"("Error In"=w707, "arg"=w705) -> ("Error Out"=w704:errorcluster[])  [unwired: 9 in]
      }
      frame "set" {
        n375 = call "LtaSet.vi"("Error In"=w717, "Data"=w716) -> ("Error Out"=w715:errorcluster[])  [unwired: 8 in, 1 out]
        n376 = call "Enqueue.vi"("ErrorArray"=w715, "Msg"="UpdateFrontPanel") -> ("ErrorArray"=w714:errorcluster[])  [unwired: 9 in]
      }
      frame "run" {
        n377 = call "StartAll.vi"("Error In"=w722) -> ("Error Out"=w720:errorcluster[], "BC_AppInfo"=w719:T41)  [unwired: 9 in]
        n378 = Empty Array?(array=w720) -> (empty?=w721:bool)
        n379 = case shown="True" w721 {
          tunnel: [w723 w735] -> w718
          tunnel: w720 -> [w723 w731]
          tunnel: w719 -> [_ w729]
          frame False {
          }
          frame True {
            # "There is only one App Module"
            n380 = call "WriteBcAppInfoRequest.vi"("InputData"=w729, "ModuleID"=-1) -> ("error out"=w732:errorcluster)  [unwired: 9 in]
            n381 = call <userlib>:"AddError.vi"("Severity"="Abort", "Priority"=u8 3, "ErrorArray"=w731, "error in (no error)"=w732) -> ("ErrorArray"=w727:errorcluster[])  [unwired: 6 in, 1 out]
            n382 = call "Enqueue.vi"("Priority (f)"=TRUE, "ErrorArray"=w727, "Msg"="LtaRunComplete") -> ("ErrorArray"=w726:errorcluster[])  [unwired: 8 in]
            n383 = call "Enqueue.vi"("Priority (f)"=TRUE, "ErrorArray"=w726, "Msg"="RunAppScript") -> ("ErrorArray"=w735:errorcluster[])  [unwired: 8 in]
          }
        }
      }
      frame "RunAppScript" {
        # "There is only one instance of the App so all buses point to it."
        n384 = call "GetSetFrameworkData.vi"() -> ("clFrameworkData Out"=w753:T30)  [unwired: 11 in]
        n385 = Unbundle By Name(w753) -> ("BusClassInstances"=w754:refnum<class "Bus.lvclass">[])
        n386 = Index Array(array=w754, index=0) -> (element=w749:refnum<class "Bus.lvclass">)
        n387 = call "RunScript.vi"("ErrorArray"=w750, "Script"=string[] ["ReadAppPluginPath", "ReadOutToFilePluginPath", "Stop"], "Bus"=w749) -> ("ErrorArray"=w743:errorcluster[], "Data out"=w747:variant, "Bus"=w744:refnum<class "Bus.lvclass">)  [unwired: 6 in]
        n388 = Variant To Data(type=T32 {"BusNumber"=0, "EvtPluginINIFilePath"=path "", "EvtParams"=[], "EvtConfig"={"UTC Time 0"=timestamp(0 s since 1904-01-01), "Nominal Frequency"=60, "Reporting Rate"=60, "Fsamp"=960, "PosSeq"=FALSE}, "Start Time"=0.0, "End Time"=0.0, "PmuImpairPluginINIFilePath"=path "", "PmuImpairParams "=[["960"], ["8.19"], ["164"]], "PmuImpairConfig"={"FilterType"="", "bPosSeq"=TRUE}, "NetImpPluginINIFilePath"=path "", "NetImpParams"=[], "FlagImpPluginINIFilePath"=path "", "FlagImpParams"=[], "EvtReportArray"=[], "EventSignalArray"=[], "ImpairReportArray"=[], "NetworkTime"=[], "PktLoss"=[], "FlagImpArray"=[], "OutputToFilePluginINIFilePath"=path "", "Output File Path"=path "", "clConfigOptions"={"TIME_BASE"=1000000, "STN"="Bus_1", "IDCODE"=0, "rdoPolRect"=enum."Rectangular", "rdoFloatInt"=enum."Float", "PHUNIT"=1000000, "rdoFreqDfreq"=enum."Float", "CHNAM"=["VA", "VB", "VC", "V+", "IA", "IB", "IC", "I+"], "chkCfg2Prefix"=TRUE}, "AppPluginINIFilePath"=path "", "AppConfig"=variant, "AppOutput"=variant} ("clBusData"), Variant=w747) -> (data=w745:T32, error out=w742:errorcluster)  [unwired: 1 in]
        n389 = Unbundle By Name(w745) -> ("AppPluginINIFilePath"=w739:path, "OutputToFilePluginINIFilePath"=w738:path)
        n390 = call <userlib>:"AddError.vi"("ErrorArray"=w743, "error in (no error)"=w742) -> ("ErrorArray"=w741:errorcluster[])  [unwired: 8 in, 1 out]
        n391 = Empty Array?(array=w741) -> (empty?=w740:bool)
        n392 = Build Array(w739, w738) -> (w737:path[])
        n393 = case shown="True" w740 {
          tunnel: [w755 w762] -> w752
          tunnel: w744 -> [_ w761]
          tunnel: w741 -> [w755 w760]
          tunnel: w737 -> [_ w757]
          frame False {
          }
          frame True {
            n394 = for {
              shift-right: [w767] -> w763
              shift-left: w760 -> [w766]
              tunnel: w757 -> [w765] mode=indexing
              tunnel: [w764] -> w756 mode=concatenating
              n395 = call "GetScriptFromIniFile.vi"("ErrorArray"=w766, "Path"=w765) -> ("ErrorArray"=w767:errorcluster[], "Script"=w764:string[])  [unwired: 8 in]
            }
            n396 = Build Array (concatenate)(w756, string[] ["Stop"] ("element")) -> (w758:string[])
            n397 = call "RunScript.vi"("ErrorArray"=w763, "Script"=w758, "Bus"=w761) -> ("ErrorArray"=w762:errorcluster[])  [unwired: 6 in, 2 out]
          }
        }
      }
      frame "GetAppOutput" {
        # "There is only one instance of the App so all buses point to it."
        n398 = call "GetSetFrameworkData.vi"() -> ("clFrameworkData Out"=w776:T30)  [unwired: 11 in]
        n399 = Unbundle By Name(w776) -> ("BusClassInstances"=w777:refnum<class "Bus.lvclass">[])
        n400 = Index Array(array=w777, index=0) -> (element=w774:refnum<class "Bus.lvclass">)
        n401 = property class="Bus.lvclass"(reference=w774) -> ("Accessors:AppModuleID"=w773:i32)  [unwired: 1 in, 2 out]
        n402 = call "GetAppOutputRequest.vi"("ModuleID"=w773) -> ("error out"=w771:errorcluster)  [unwired: 10 in]
        n403 = call <userlib>:"AddError.vi"("Severity"="Abort", "Priority"=u8 3, "ErrorArray"=w772, "error in (no error)"=w771) -> ("ErrorArray"=w768:errorcluster[])  [unwired: 6 in, 1 out]
      }
      frame "LtaRunComplete" {
        n404 = call "Transmitter.vi"("ErrorArray"=w780, "Command"="LtaRunComplete") -> ("ErrorArray"=w779:errorcluster[])  [unwired: 8 in, 1 out]
      }
      frame "Visualize" {
        n405 = call "dlgSelectVisApps.vi"("Error In"=w781) -> ("Error Out"=w782:errorcluster[])  [unwired: 10 in]
      }
      frame "ClientError" {
        n406 = Variant To Data(type="", Variant=w784) -> (data=w793:string)  [unwired: 1 in, 1 out]
        n407 = Unflatten From XML(xml string=w793, type=errorcluster {"status"=FALSE, "code"=0, "source"=""} ("error constant")) -> (value=w788:errorcluster, error out=w790:errorcluster)  [unwired: 1 in]
        n408 = call <userlib>:"AddError.vi"("Severity"="Abort", "Priority"=u8 3, "ErrorArray"=w785, "error in (no error)"=w790) -> ("ErrorArray"=w789:errorcluster[])  [unwired: 6 in, 1 out]
        n409 = Build Array (concatenate)(w788, w789) -> (w783:errorcluster[])
      }
      frame "Error" {
        n410 = Variant To Data(type=errorcluster[] [], Variant=w800) -> (data=w798:errorcluster[])  [unwired: 1 in, 1 out]
        n411 = call <userlib>:"ParseErrors.vi"("ErrorArray"=w798) -> ("ErrorArray"=w797:errorcluster[])  [unwired: 8 in, 2 out]
        n412 = for {
          tunnel: w797 -> [w803] mode=indexing
          tunnel: [w801] -> w795 mode=concatenating
          n413 = call <userlib>:"GeneralHandler.vi"("error in (no error)"=w803) -> ("Severity"=w809:string, "Stop"=w807:bool, "Abort"=w806:bool, "Continue"=w808:bool)  [unwired: 7 in]
          n414 = Unbundle By Name(w803) -> ("source"=w802:string)
          n415 = Build Array(w808, w806, w807) -> (w804:bool[])
          n416 = Boolean Array To Number(Boolean array=w804) -> (number=w805:u32)
          n417 = case shown="1" w805 {
            tunnel: w809 -> [_ w811 w818 w827]
            tunnel: [_ _ w817 w826] -> w801
            tunnel: w802 -> [_ w810 _ _]
            frame 0, Default {
              # "No dialogue button pressed."
            }
            frame 1 {
              # "Continue button pressed."
              n418 = case shown="Default" w811 {
                tunnel: w810 -> [_ w812]
                frame Default {
                  # "Let the Framework continue."
                }
                frame "Log" {
                  # "Write to log file in this case?"
                  n419 = Get Date/Time String(want seconds? (F)=TRUE) -> (time string=w815:string)  [unwired: 2 in, 1 out]
                  n420 = call <vilib>:"Space Constant.vi"() -> ("String"=w814:string)
                  n421 = Concatenate Strings(w815, w814, w812, "\r\n") -> ()  [unwired: 1 out]
                }
              }
            }
            frame 2 {
              # "Abort button pressed."
              n422 = case shown="Default" w818 {
                tunnel: [w824] -> w817
                frame Default {
                  # "Flush queue if aborted."
                  n423 = call "ObtainMsgQueue.vi"() -> ("ErrorArray"=w822:errorcluster[], "QueRef"=w825:T44)  [unwired: 10 in]
                  n424 = Flush Queue(queue=w825) -> (error out=w823:errorcluster)  [unwired: 1 in, 2 out]
                  n425 = call <userlib>:"AddError.vi"("Severity"="Critical" ("String"), "Priority"=u8 1, "ErrorArray"=w822, "error in (no error)"=w823) -> ("ErrorArray"=w824:errorcluster[], "error out"=w819:errorcluster)  [unwired: 6 in]
                  n426 = call <vilib>:"Clear Errors.vi"("error in (no error)"=w819) -> ()  [unwired: 5 in, 2 out]
                }
              }
            }
            frame 4 {
              # "Stop button pressed."
              n427 = case shown="Default" w827 {
                tunnel: [w828] -> w826
                frame Default {
                  n428 = call "StopRequest.vi"() -> ("ErrorArray Out"=w828:errorcluster[])  [unwired: 11 in]
                }
              }
            }
          }
        }
        n429 = call <userlib>:"ClearErrors.vi"() -> ("ErrorArray"=w796:errorcluster[])  [unwired: 11 in]
        n430 = Build Array (concatenate)(w795, w796) -> (w794:errorcluster[])
      }
      frame "Stop" {
        w833 = TRUE
        # "Remove all buses (close all modules), save the front panel control data, and stop the QMH Loop."
        n431 = call "RemoveBus.vi"("Remove All? (F)"=TRUE, "ErrorArray In"=w834) -> ("ErrorArray Out"=w832:errorcluster[])  [unwired: 9 in]
        n432 = call "RemoveApp.vi"("ErrorArray In"=w832) -> ("ErrorArray Out"=w831:errorcluster[])  [unwired: 10 in]
        n433 = call "RemoveOutToFile.vi"("ErrorArray In"=w831) -> ("ErrorArray Out"=w830:errorcluster[])  [unwired: 10 in]
        n434 = call "FrontPanelToIni.vi"("ErrorArray In"=w830) -> ("ErrorArray Out"=w829:errorcluster[])  [unwired: 10 in]
        n435 = call "StopProg.vi"("Stop (f)"=w833) -> ()  [unwired: 10 in, 1 out]
      }
    }
    n436 = call "EnqueueError.vi"("ErrorArray"=w654) -> ("ErrorArray"=w655:errorcluster[])  [unwired: 10 in]
  }
  n437 = while {
    shift-right: [w836] -> _
    shift-left: w23 -> [w841]
    stop <- w838 stop-if-true
    # "TCP Receive Loop (LV-PY)"
    n438 = call "Listener.vi"("ErrorArray"=w841) -> ("ErrorArray"=w840:errorcluster[], "Accepted?"=w839:bool)  [unwired: 9 in]
    n439 = case shown="True" w839 {
      tunnel: w840 -> [w842 w844]
      tunnel: [w842 w843] -> w837
      frame False {
      }
      frame True {
        n440 = while {
          tunnel: w844 -> [w854]
          tunnel: [w845] -> w843
          stop <- w851 stop-if-true
          n441 = call "Receiver.vi"("ErrorArray"=w854) -> ("ErrorArray"=w849:errorcluster[], "XMLData"=w848:string, "Command"=w847:string, "error out"=w852:errorcluster, "bytes_read"=w850:i32)  [unwired: 6 in]
          n442 = call "StopProg.vi"() -> ("Stop?"=w853:bool)  [unwired: 11 in]
          n443 = case shown="1, Default" w850 {
            tunnel: w849 -> [w855 w859]
            tunnel: w848 -> [_ w858]
            tunnel: w847 -> [_ w857]
            tunnel: [w855 w856] -> w846
            frame 0 {
            }
            frame 1, Default {
              n444 = To Variant(anything=w858) -> (Variant=w860:variant)
              n445 = call "Enqueue.vi"("ErrorArray"=w859, "Data"=w860, "Msg"=w857) -> ("ErrorArray"=w856:errorcluster[])  [unwired: 8 in]
            }
          }
          n446 = Or(x=w852, y=w853) -> (x .or. y?=w851:bool)
          n447 = call "EnqueueError.vi"("ErrorArray"=w846) -> ("ErrorArray"=w845:errorcluster[])  [unwired: 10 in]
        }
      }
    }
    n448 = call "StopProg.vi"() -> ("Stop?"=w838:bool)  [unwired: 11 in]
    n449 = call "EnqueueError.vi"("ErrorArray"=w837) -> ("ErrorArray"=w836:errorcluster[])  [unwired: 10 in]
  }
